vi "Omniax_mDrive_XY_MM_BR_RES.vi"() -> ()   [LabVIEW 2009]
uses:
  <vilib>/Instr/_visa.llb/VISA Configure Serial Port (Instr).vi
panel:
  out "Reset X Motor Steps":i32
  in  "Rese X Position mm":dbl
  out "X Backlash corr":bool
  out "X  in Motion":bool
  out "X Scan":bool
  out "X  in Range":bool
  out "X Step PV":i32 max=2000
  out "X Position mm PV":dbl
  out "X scan steps/sec MV step/sec":i32
  in  "X Scan set":bool
  in  "X Scan Velocity SP mm/sec":dbl
  in  "X Scan Length SP mm":dbl
  in  "X Move Set":bool
  out "X Velocity MV mm/sec":dbl
  in  "X Velocity SP mm/sec":dbl
  in  "X Position SP mm":dbl
  out "X Position MV mm":dbl
  out "X Scan velocity MV mm/sec":dbl format="%#_6f"
  out "X Scan length MV mm":dbl
  in  "X Scan Length SP steps":i32 min=-460800 max=460800 step=100
  in  "X Scan OK":bool
  in  "X Velocity SP step/sec":i32 min=1 max=102400
  in  "X Scan Velocity SP steps/sec":i32=1 min=1 max=102400 step=1
  in  "X Go":bool
  in  "X Step SP":i32=-20000 min=-460800 max=460800 step=500
  out "X Backlash steps/sec":i32
  out "X Backlash":i32
  out "X Holding Current %":i32
  out "X Run Current %":i32
  out "X offset mm":dbl
  out "X mm/rev":dbl
  out "X steps/rev":u32
  out "X MAXPOS":i32=-34296
  out "X MINPOS":i32=-94296
  out "X COM PORT":refnum<visa-resource-name>="COM5"
  out "Y Backlash corr":bool
  in  "Y Scan set":bool
  in  "Y Scan Velocity SP mm/sec":dbl
  in  "Y Scan Length SP mm":dbl
  in  "Y Move Set":bool
  out "Y Backlash steps/sec":i32
  out "Y Backlash":i32
  out "Y in Motion":bool
  in  "Reset":bool
  out "Reset Y Motor Steps":i32
  in  "Reset Y Position mm":dbl
  out "Y Velocity MV mm/sec":dbl
  in  "Y Velocity SP mm/sec":dbl
  in  "Y Position SP mm":dbl
  out "Y Position MV mm":dbl
  out "Y Holding Current %":i32
  out "Y Run Current %":i32
  out "Y Scan velocity MV mm/sec":dbl format="%#_6f"
  out "Y Scan length MV mm":dbl
  in  "Scan Cancel":bool
  out "Y Position mm PV":dbl
  out "Y offset mm":dbl
  out "Y mm/rev":dbl
  out "Y steps/rev":u32
  out "Y scan steps/sec MV step/sec":i32
  in  "Y Scan Length SP steps":i32 min=-460800 max=460800 step=100
  out "Y Scan":bool
  in  "Y Scan OK":bool
  in  "Scan Go":bool
  in  "Y Velocity SP step/sec":i32 min=1 max=102400
  in  "Y Scan Velocity SP steps/sec":i32=1 min=1 max=102400 step=1
  in  "Stop":bool
  out "Y in Range":bool
  out "Y Step PV":i32 max=2000
  in  "Y Go":bool
  in  "Y Step SP":i32=-20000 min=-460800 max=460800 step=500
  out "Y MINPOS":i32=-94296
  out "Y MAXPOS":i32=-34296
  out "Y COM PORT":refnum<visa-resource-name>="COM5"
  # "LM"
  # "MV"
  # "BL"
  # "SC"
  # "MX"
  # "MY"
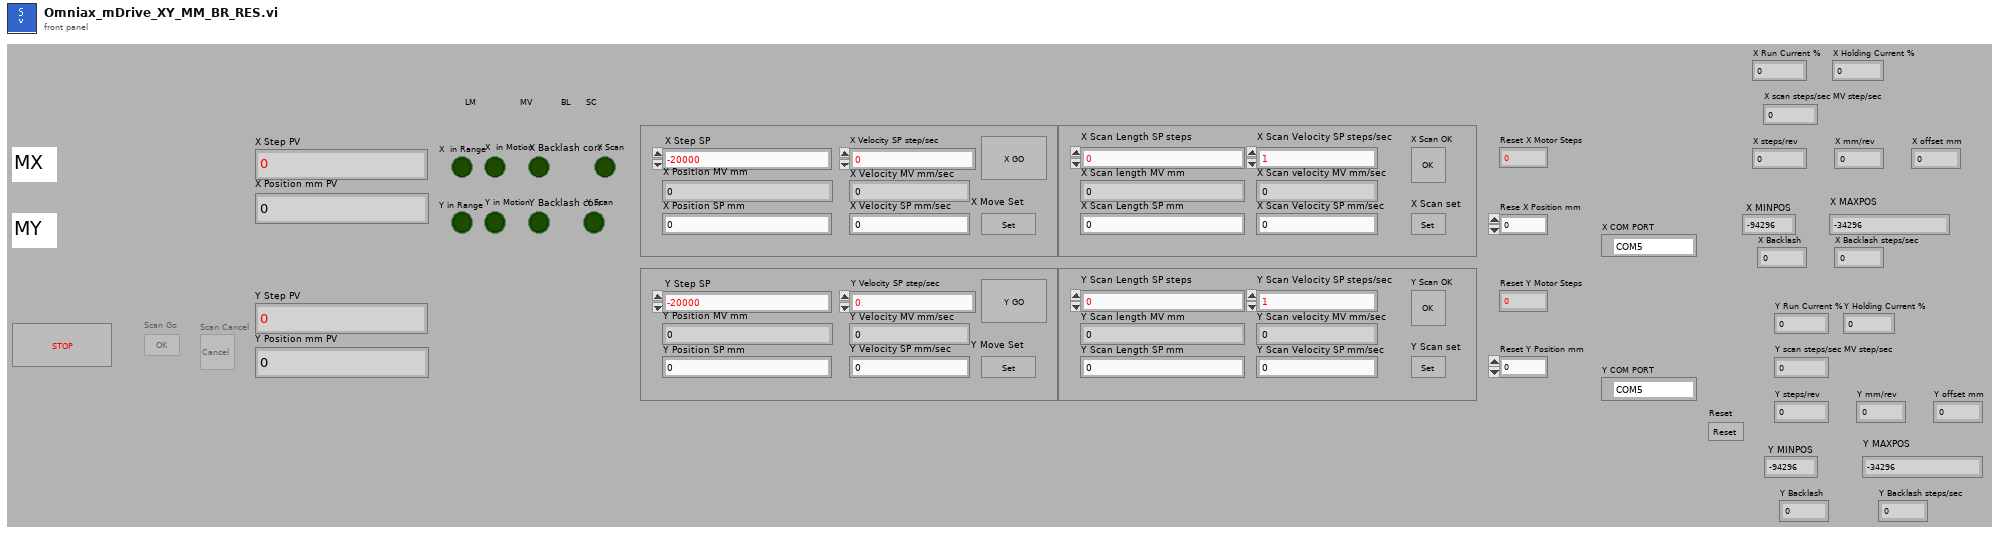
[diagram p1: front panel]
types:
  T1 = enum8{"Enabled", "Disabled", "Disabled and Grayed Out"}
  T2 = enum16{"Stop", "Reset", "Run Current", "Holding Current", "Accel Rate", "Decel Rate", "Move to Relative Position", "Move to Absolute Position", "Echo Mode", "Print Parameter", "Send String", "Microstep Resolution", "Set Current Position", "Max Velocity"}
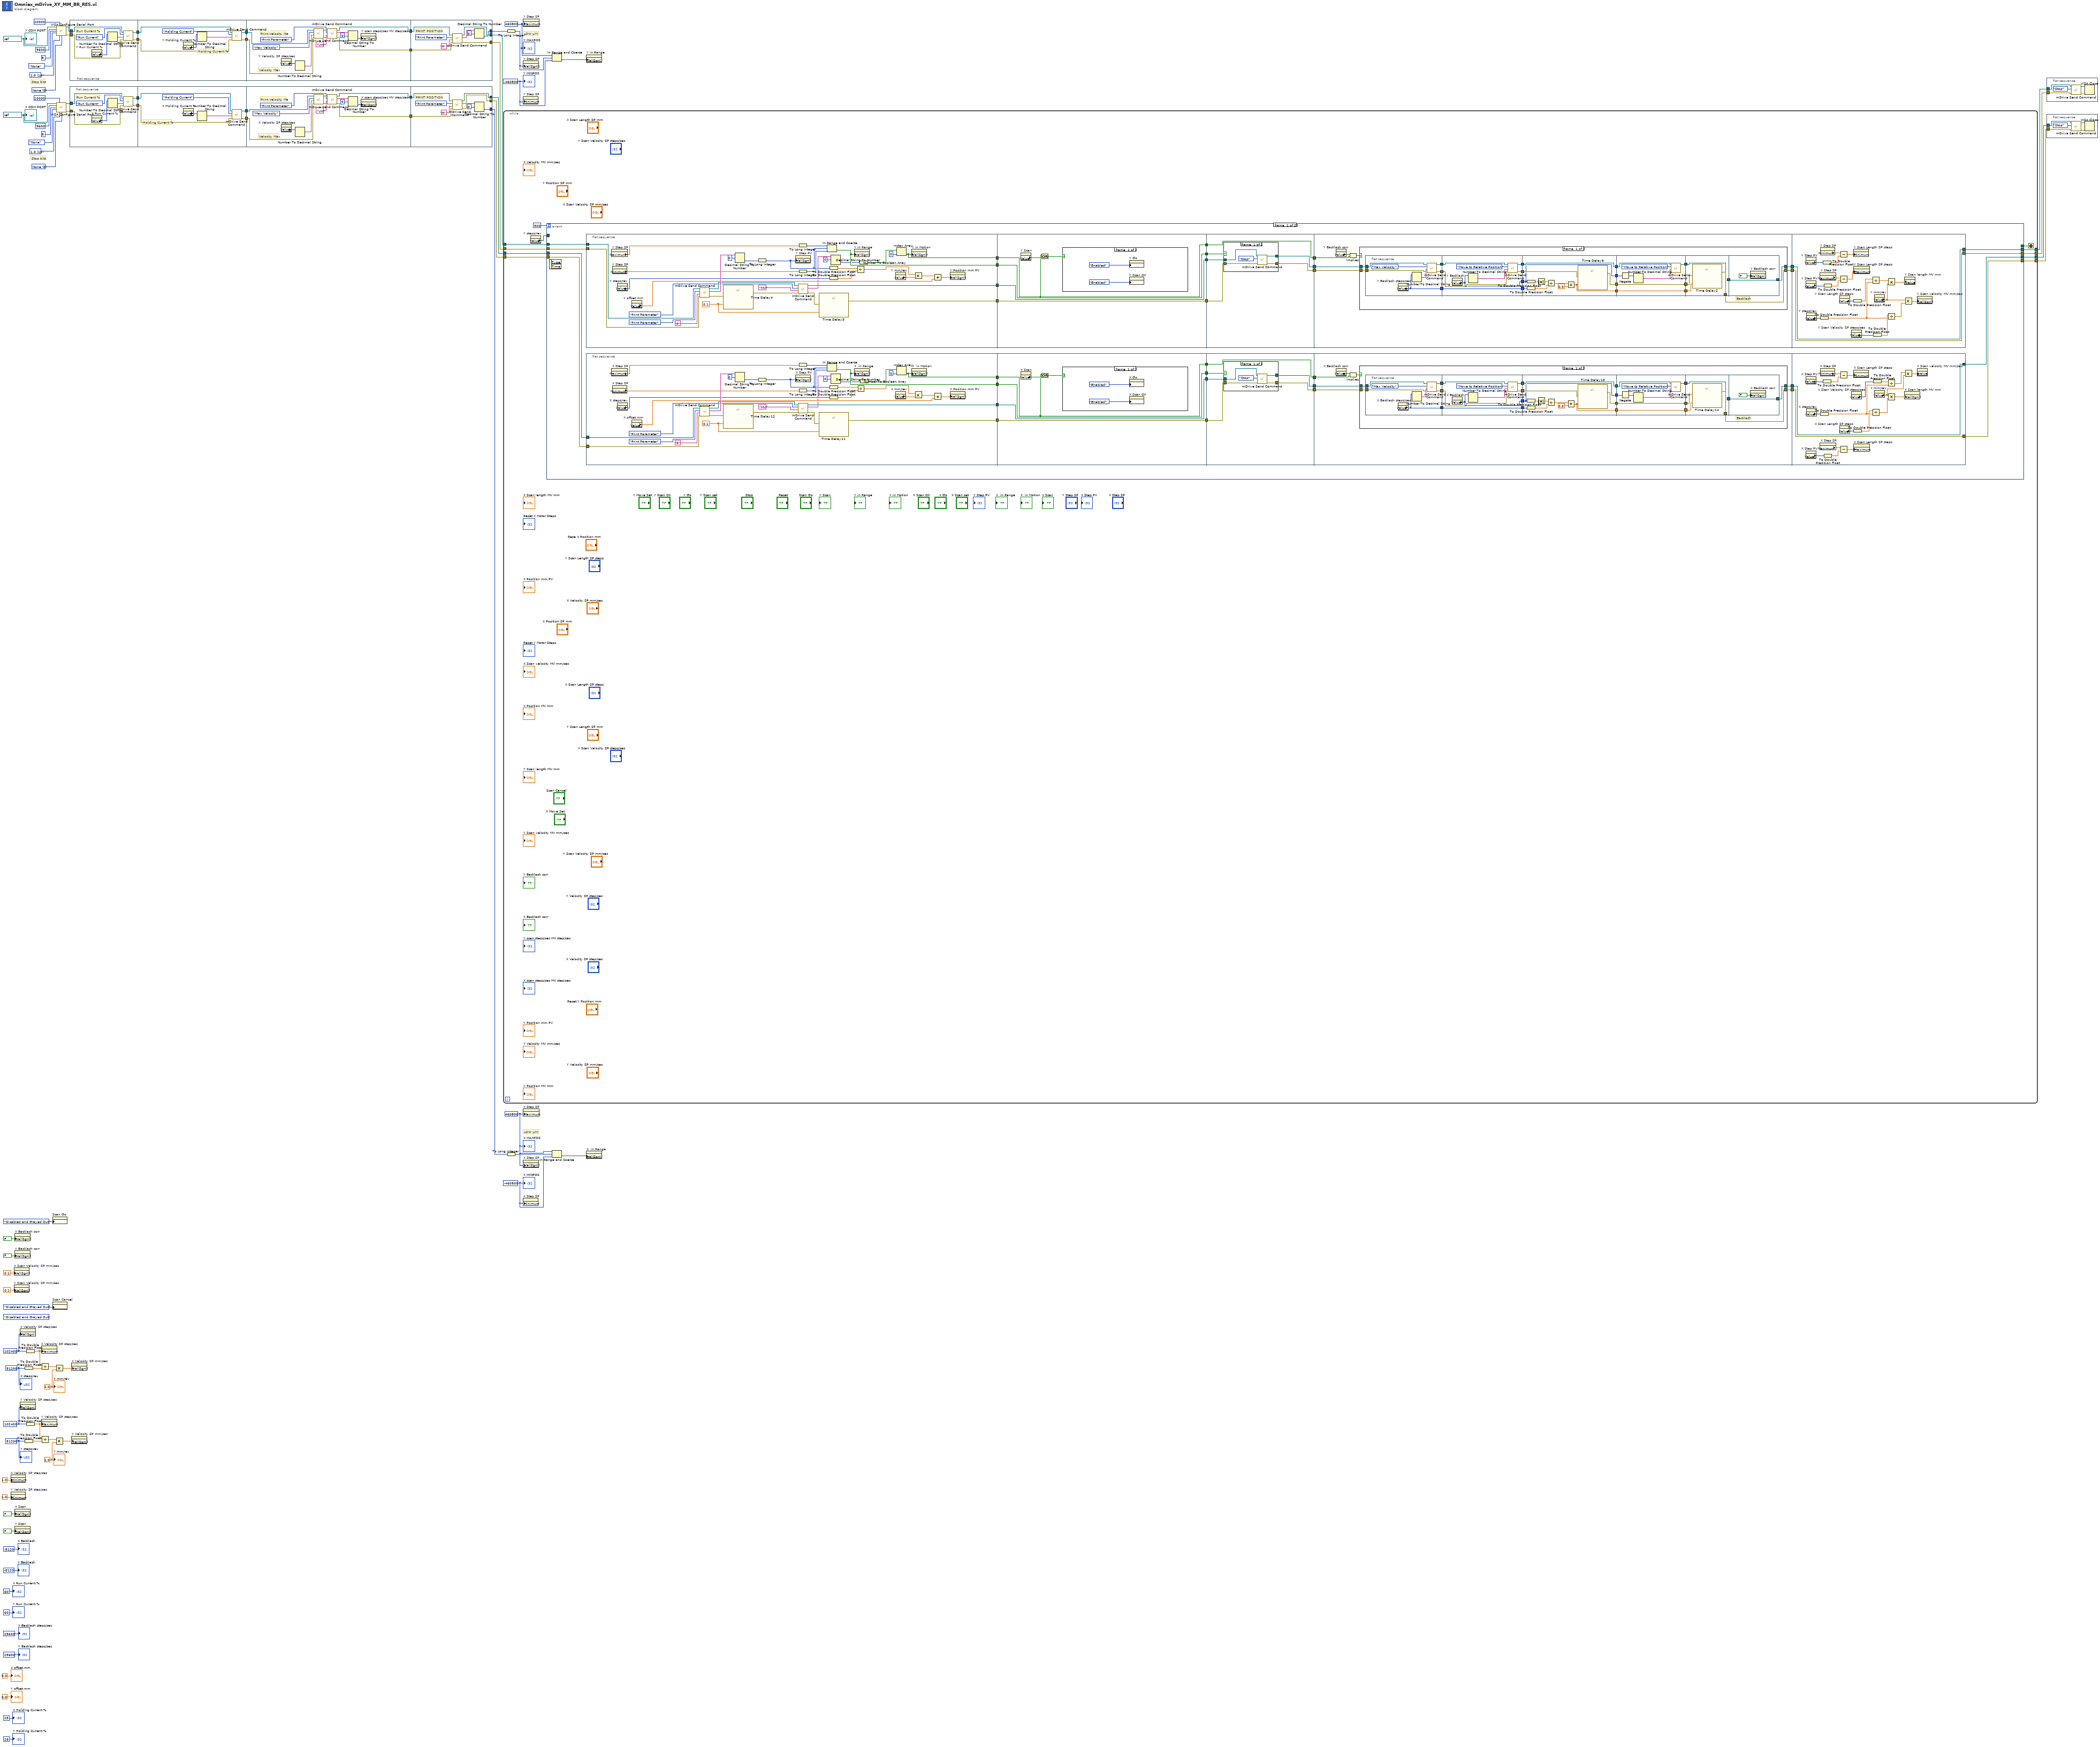
[diagram p0: block diagram]
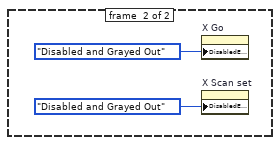
[diagram p2: hidden frame]
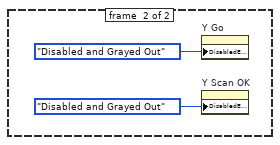
[diagram p5: hidden frame]
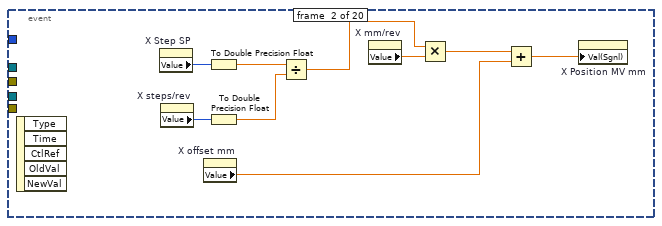
[diagram p8: hidden frame]
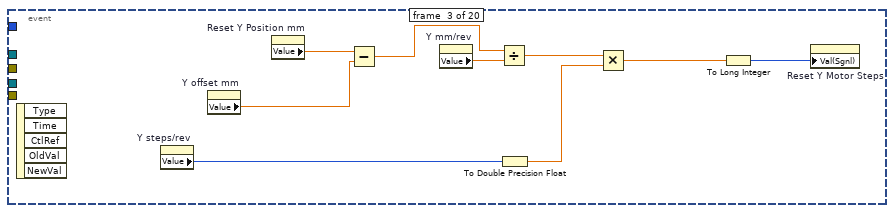
[diagram p9: hidden frame]
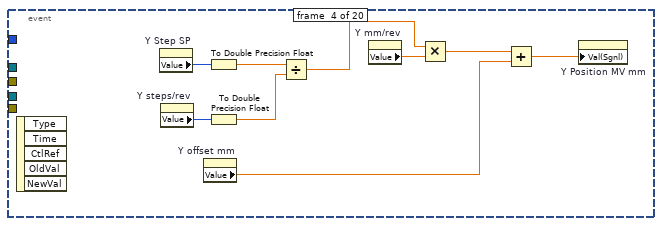
[diagram p10: hidden frame]
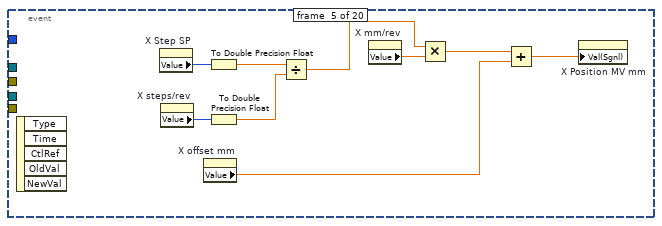
[diagram p11: hidden frame]
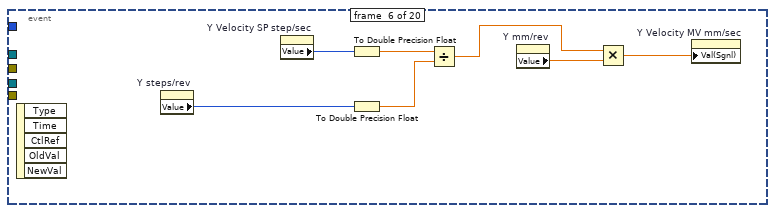
[diagram p12: hidden frame]
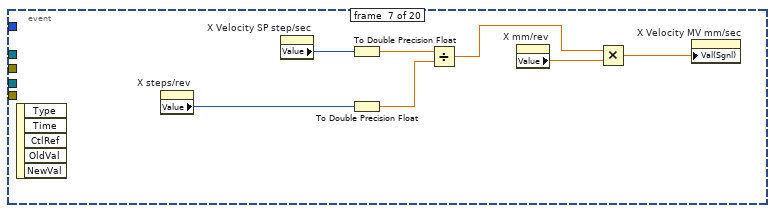
[diagram p13: hidden frame]
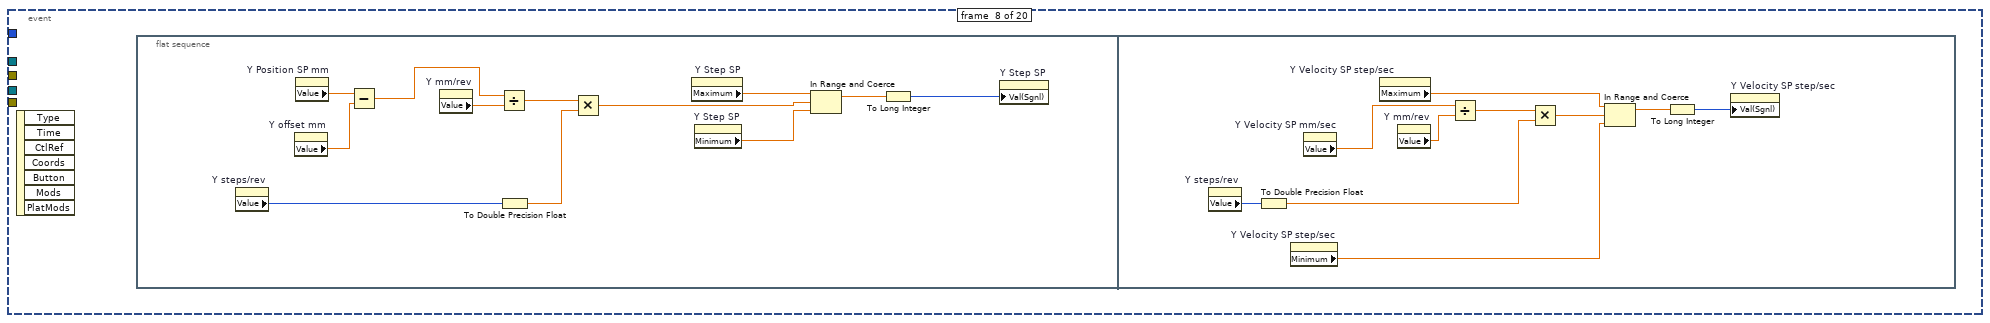
[diagram p14: hidden frame]
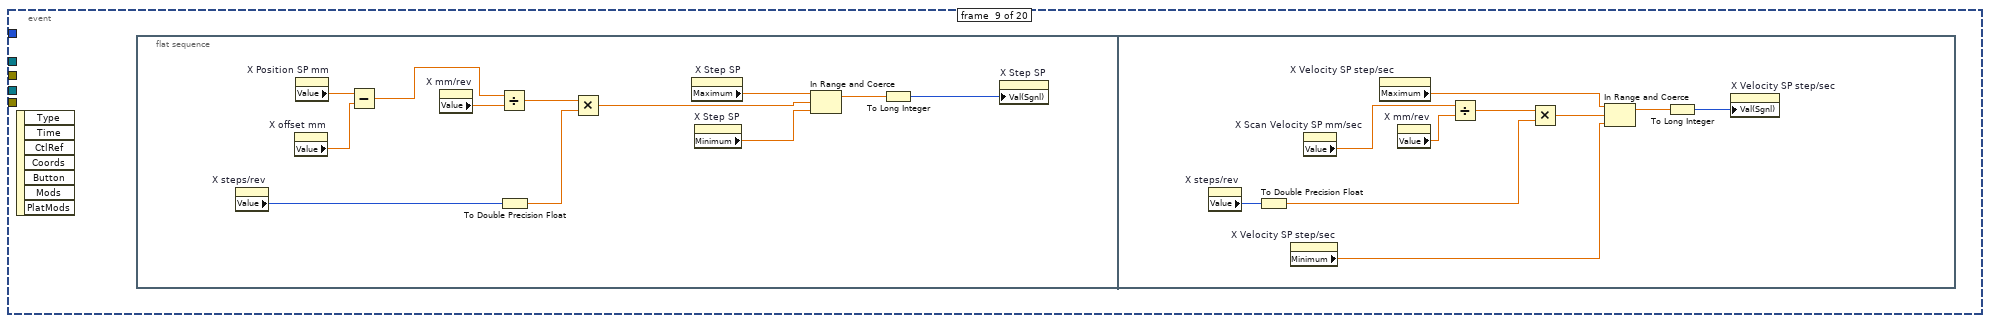
[diagram p15: hidden frame]
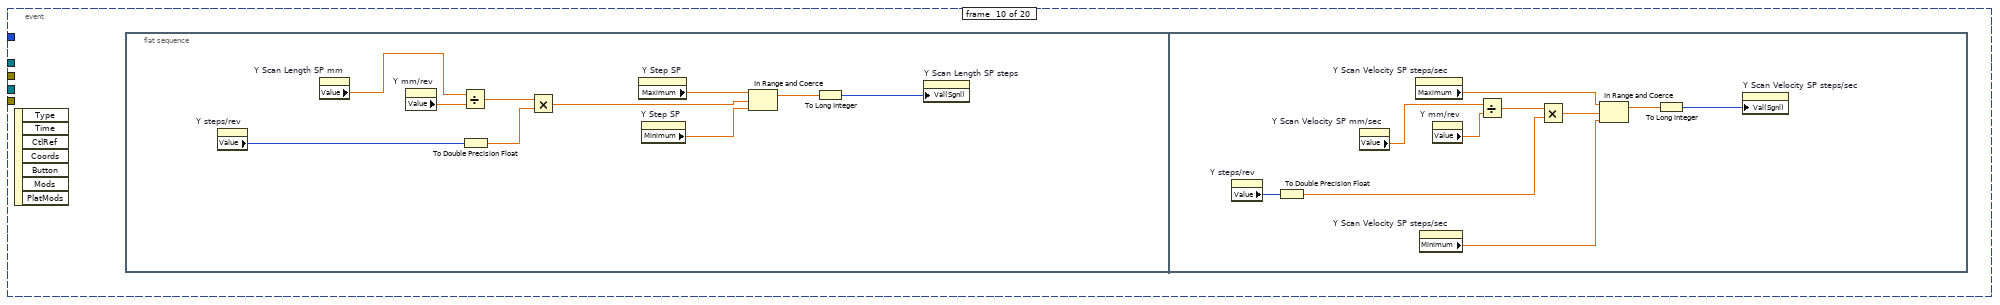
[diagram p16: hidden frame]
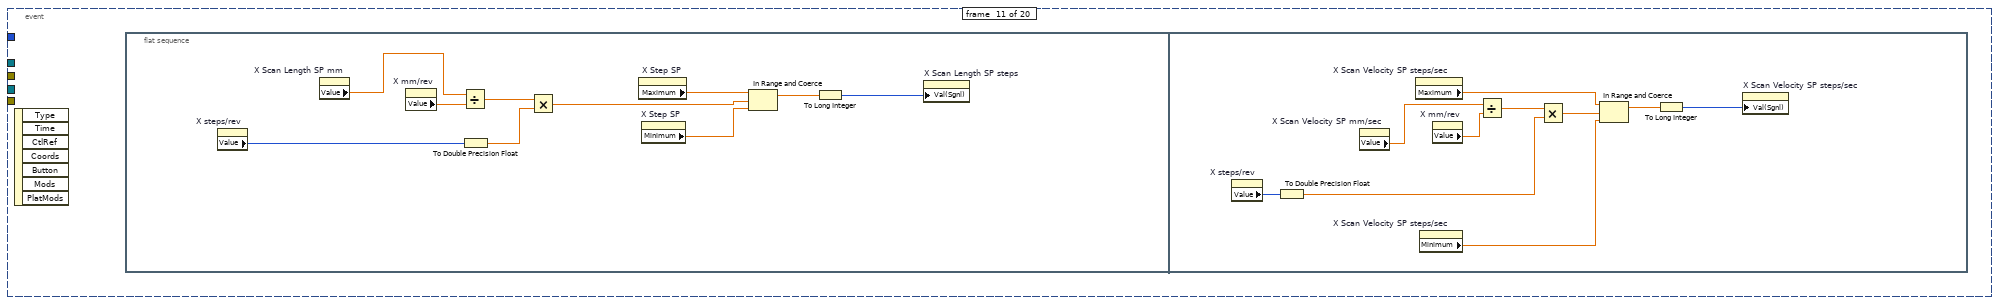
[diagram p17: hidden frame]
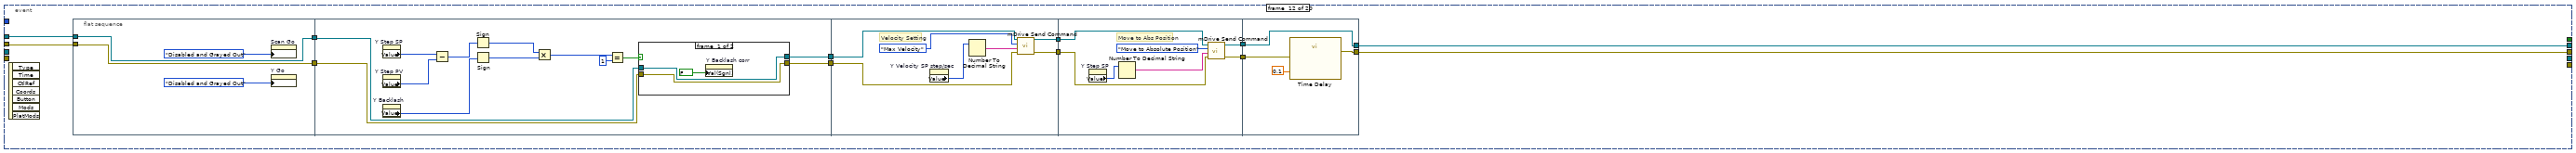
[diagram p18: hidden frame]
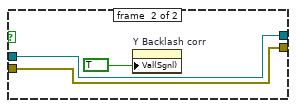
[diagram p19: hidden frame]
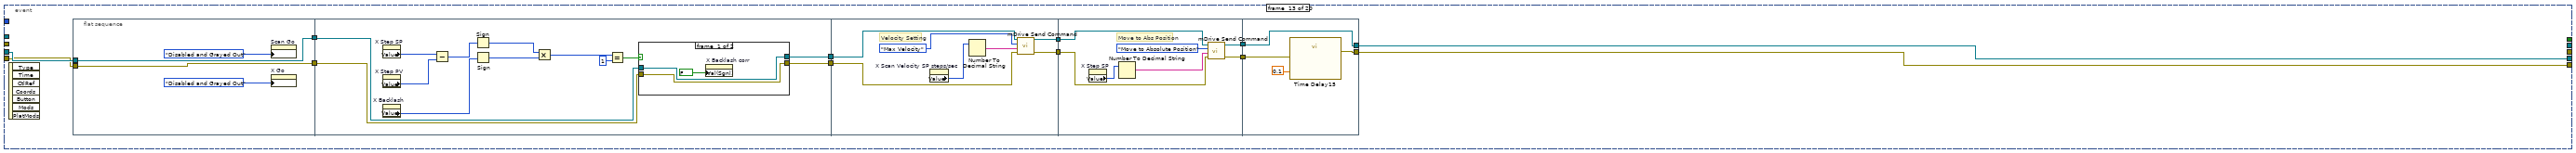
[diagram p20: hidden frame]
diagram:
  (unwired) T1."Disabled and Grayed Out" ("Disabled")
  w13 = 1.0 ("MM/rev")
  w10 = u32 51200 ("step/rev")
  w15 = 102400 ("Value (Signaling)")
  w25 = -460800 ("lower limit")
  w24 = 460800 ("upper limit")
  w28 = refnum<visa-resource-name> "COM8" ("COM PORT")
  w30 = u16 0 items=["None", "XON/XOFF", "RTS/CTS", "XON/XOFF & RTS/CTS", "DTR/DSR", "XON/XOFF & DTR/DSR"] ("flow control (0:none)")
  w31 = u16 10 items=["1.0"=10, "1.5"=15, "2.0"=20] ("stop bits (10: 1 bit)")
  w49 = 1.0 ("MM/rev")
  w46 = u32 51200 ("step/rev")
  w51 = 102400 ("Value (Signaling)")
  w69 = -460800 ("lower limit")
  w68 = 460800 ("upper limit")
  w76 = refnum<visa-resource-name> "COM9" ("COM PORT")
  w78 = u16 0 items=["None", "XON/XOFF", "RTS/CTS", "XON/XOFF & RTS/CTS", "DTR/DSR", "XON/XOFF & DTR/DSR"] ("flow control (0:none)")
  w79 = u16 10 items=["1.0"=10, "1.5"=15, "2.0"=20] ("stop bits (10: 1 bit)")
  # "LOW LIM"
  # "Stop bits"
  # "LOW LIM"
  # "Stop bits"
  n1 = property on="X Velocity SP step/sec" class="DigNum (strict)"("Minimum"=1.0 ("Data Entry Limits:Minimum")) -> ()  [unwired: 2 in, 2 out]
  n2 = property on="Y Velocity SP step/sec" class="DigNum (strict)"("Minimum"=1.0 ("Data Entry Limits:Minimum")) -> ()  [unwired: 2 in, 2 out]
  n3 = property on="X Scan Velocity SP mm/sec" class="DigNum (strict)"("Val(Sgnl)"=0.1 ("Value (Signaling)")) -> ()  [unwired: 2 in, 2 out]
  n4 = property on="Y Scan Velocity SP mm/sec" class="DigNum (strict)"("Val(Sgnl)"=0.1 ("Value (Signaling)")) -> ()  [unwired: 2 in, 2 out]
  n5 = property on="X Backlash corr" class="Bool (strict)"("Val(Sgnl)"=FALSE ("Value (Signaling)")) -> ()  [unwired: 2 in, 2 out]
  n6 = property on="Y Backlash corr" class="Bool (strict)"("Val(Sgnl)"=FALSE ("Value (Signaling)")) -> ()  [unwired: 2 in, 2 out]
  n7 = property on="X Scan" class="Bool (strict)"("Val(Sgnl)"=FALSE ("Value (Signaling)")) -> ()  [unwired: 2 in, 2 out]
  n8 = property on="Y Scan" class="Bool (strict)"("Val(Sgnl)"=FALSE ("Value (Signaling)")) -> ()  [unwired: 2 in, 2 out]
  n9 = property on="X Velocity SP step/sec" class="DigNum (strict)"("Val(Sgnl)"=w15) -> ()  [unwired: 2 in, 2 out]
  n10 = property on="Y Velocity SP step/sec" class="DigNum (strict)"("Val(Sgnl)"=w51) -> ()  [unwired: 2 in, 2 out]
  n11 = To Double Precision Float(number=w10) -> (double precision float=w11:dbl)
  n12 = To Double Precision Float(number=w46) -> (double precision float=w47:dbl)
  n13 = To Double Precision Float(number=w15) -> (double precision float=w9:dbl)
  n14 = To Double Precision Float(number=w51) -> (double precision float=w45:dbl)
  n15 = Divide(x=w9, y=w11) -> (x/y=w14:dbl)
  n16 = Divide(x=w45, y=w47) -> (x/y=w50:dbl)
  n17 = property on="X Velocity SP step/sec" class="DigNum (strict)"("Maximum"=w9) -> ()  [unwired: 2 in, 2 out]
  n18 = property on="Y Velocity SP step/sec" class="DigNum (strict)"("Maximum"=w45) -> ()  [unwired: 2 in, 2 out]
  n19 = property on="Scan Go" class="Bool"("DisabledEnum"=T1."Disabled and Grayed Out" ("Disabled")) -> ()  [unwired: 2 in, 2 out]
  n20 = property on="Scan Cancel" class="Bool"("DisabledEnum"=T1."Disabled and Grayed Out" ("Disabled")) -> ()  [unwired: 2 in, 2 out]
  n21 = Multiply(x=w14, y=w13) -> (x*y=w12:dbl)
  n22 = Multiply(x=w50, y=w49) -> (x*y=w48:dbl)
  n23 = call-poly "VISA Configure Serial Port"("VISA resource name"=w76, "timeout (10sec)"=u32 10000, "baud rate (9600)"=u32 9600, "data bits (8)"=u16 8, "parity (0:none)"=enum16{"None", "Odd", "Even", "Mark", "Space"}."None", "stop bits (10: 1 bit)"=w79, "flow control (0:none)"=w78) -> ("VISA resource name out"=w64:refnum<visa-resource-name>, "error out"=w63:errorcluster)  [unwired: 7 in]
  n24 = call-poly "VISA Configure Serial Port"("VISA resource name"=w28, "timeout (10sec)"=u32 10000, "baud rate (9600)"=u32 9600, "data bits (8)"=u16 8, "parity (0:none)"=enum16{"None", "Odd", "Even", "Mark", "Space"}."None", "stop bits (10: 1 bit)"=w31, "flow control (0:none)"=w30) -> ("VISA resource name out"=w22:refnum<visa-resource-name>, "error out"=w21:errorcluster)  [unwired: 7 in]
  n25 = flat-sequence {
    tunnel: w63 -> [w89]
    tunnel: w64 -> [w87]
    tunnel: [w86] -> w58
    tunnel: [w88] -> w56
    tunnel: w58 -> [w96]
    tunnel: [w95] -> w57
    tunnel: w56 -> [w93]
    tunnel: [w94] -> w55
    tunnel: [w106] -> w66
    tunnel: [w107] -> w65
    tunnel: w57 -> [w105]
    tunnel: w55 -> [w104]
    tunnel: [w119] -> w75
    tunnel: [w118] -> w74
    tunnel: [w113] -> w67
    tunnel: w66 -> [w117]
    tunnel: w65 -> [w116]
    frame #0 {
      # "Run Current %"
      n26 = property on="Y Run Current %" class="DigNum (strict)"() -> ("Value"=w84:i32)  [unwired: 2 in, 2 out]
      n27 = Number To Decimal String(number=w84) -> (decimal integer string=w85:string)  [unwired: 1 in]
      n28 = call "mDrive Send Command.vi"("error in (no error)"=w89, "Extra"=w85, "Command"=T2."Run Current", "VISA resource name"=w87) -> ("error out"=w88:errorcluster, "VISA resource name out"=w86:refnum<visa-resource-name>)  [unwired: 3 in, 1 out]
    }
    frame #1 {
      # "Holding Current %"
      n29 = property on="Y Holding Current %" class="DigNum (strict)"() -> ("Value"=w91:i32)  [unwired: 2 in, 2 out]
      n30 = Number To Decimal String(number=w91) -> (decimal integer string=w92:string)  [unwired: 1 in]
      n31 = call "mDrive Send Command.vi"("error in (no error)"=w93, "Extra"=w92, "Command"=T2."Holding Current", "VISA resource name"=w96) -> ("error out"=w94:errorcluster, "VISA resource name out"=w95:refnum<visa-resource-name>)  [unwired: 3 in, 1 out]
    }
    frame #2 {
      # "Print Velocity Ma"
      # "Velocity Max"
      n32 = property on="Y Velocity SP step/sec" class="DigNum (strict)"() -> ("Value"=w103:i32)  [unwired: 2 in, 2 out]
      n33 = Number To Decimal String(number=w103) -> (decimal integer string=w102:string)  [unwired: 1 in]
      n34 = call "mDrive Send Command.vi"("error in (no error)"=w104, "Extra"=w102, "Command"=T2."Max Velocity", "VISA resource name"=w105) -> ("error out"=w100:errorcluster, "VISA resource name out"=w110:refnum<visa-resource-name>)  [unwired: 3 in, 1 out]
      n35 = call "mDrive Send Command.vi"("error in (no error)"=w100, "Extra"="VM", "Command"=T2."Print Parameter", "VISA resource name"=w110) -> ("error out"=w107:errorcluster, "read buffer"=w108:string, "VISA resource name out"=w106:refnum<visa-resource-name>)  [unwired: 3 in]
      n36 = Decimal String To Number(string=w108, offset=0) -> (number=w101:i32)  [unwired: 1 in, 1 out]
      n37 = property on="Y scan steps/sec MV step/sec" class="DigNum (strict)"("Val(Sgnl)"=w101) -> ()  [unwired: 2 in, 2 out]
    }
    frame #3 {
      # "PRINT POSITION"
      n38 = call "mDrive Send Command.vi"("error in (no error)"=w116, "Extra"="P", "Command"=T2."Print Parameter", "VISA resource name"=w117) -> ("error out"=w118:errorcluster, "read buffer"=w115:string, "VISA resource name out"=w119:refnum<visa-resource-name>)  [unwired: 3 in]
      n39 = Decimal String To Number(string=w115, offset=0) -> (number=w113:i32)  [unwired: 1 in, 1 out]
    }
  }
  n40 = flat-sequence {
    tunnel: w21 -> [w126]
    tunnel: w22 -> [w124]
    tunnel: [w123] -> w40
    tunnel: [w125] -> w39
    tunnel: w40 -> [w133]
    tunnel: [w132] -> w38
    tunnel: w39 -> [w130]
    tunnel: [w131] -> w37
    tunnel: [w143] -> w36
    tunnel: [w144] -> w35
    tunnel: w38 -> [w142]
    tunnel: w37 -> [w141]
    tunnel: [w156] -> w4
    tunnel: [w155] -> w3
    tunnel: [w150] -> w23
    tunnel: w36 -> [w154]
    tunnel: w35 -> [w153]
    frame #0 {
      # "Run Current %"
      n41 = property on="X Run Current %" class="DigNum (strict)"() -> ("Value"=w121:i32)  [unwired: 2 in, 2 out]
      n42 = Number To Decimal String(number=w121) -> (decimal integer string=w122:string)  [unwired: 1 in]
      n43 = call "mDrive Send Command.vi"("error in (no error)"=w126, "Extra"=w122, "Command"=T2."Run Current", "VISA resource name"=w124) -> ("error out"=w125:errorcluster, "VISA resource name out"=w123:refnum<visa-resource-name>)  [unwired: 3 in, 1 out]
    }
    frame #1 {
      # "Holding Current %"
      n44 = property on="X Holding Current %" class="DigNum (strict)"() -> ("Value"=w128:i32)  [unwired: 2 in, 2 out]
      n45 = Number To Decimal String(number=w128) -> (decimal integer string=w129:string)  [unwired: 1 in]
      n46 = call "mDrive Send Command.vi"("error in (no error)"=w130, "Extra"=w129, "Command"=T2."Holding Current", "VISA resource name"=w133) -> ("error out"=w131:errorcluster, "VISA resource name out"=w132:refnum<visa-resource-name>)  [unwired: 3 in, 1 out]
    }
    frame #2 {
      # "Print Velocity Ma"
      # "Velocity Max"
      n47 = property on="X Velocity SP step/sec" class="DigNum (strict)"() -> ("Value"=w140:i32)  [unwired: 2 in, 2 out]
      n48 = Number To Decimal String(number=w140) -> (decimal integer string=w139:string)  [unwired: 1 in]
      n49 = call "mDrive Send Command.vi"("error in (no error)"=w141, "Extra"=w139, "Command"=T2."Max Velocity", "VISA resource name"=w142) -> ("error out"=w137:errorcluster, "VISA resource name out"=w147:refnum<visa-resource-name>)  [unwired: 3 in, 1 out]
      n50 = call "mDrive Send Command.vi"("error in (no error)"=w137, "Extra"="VM", "Command"=T2."Print Parameter", "VISA resource name"=w147) -> ("error out"=w144:errorcluster, "read buffer"=w145:string, "VISA resource name out"=w143:refnum<visa-resource-name>)  [unwired: 3 in]
      n51 = Decimal String To Number(string=w145, offset=0) -> (number=w138:i32)  [unwired: 1 in, 1 out]
      n52 = property on="X scan steps/sec MV step/sec" class="DigNum (strict)"("Val(Sgnl)"=w138) -> ()  [unwired: 2 in, 2 out]
    }
    frame #3 {
      # "PRINT POSITION"
      n53 = call "mDrive Send Command.vi"("error in (no error)"=w153, "Extra"="P", "Command"=T2."Print Parameter", "VISA resource name"=w154) -> ("error out"=w155:errorcluster, "read buffer"=w152:string, "VISA resource name out"=w156:refnum<visa-resource-name>)  [unwired: 3 in]
      n54 = Decimal String To Number(string=w152, offset=0) -> (number=w150:i32)  [unwired: 1 in, 1 out]
    }
  }
  n55 = property on="X Velocity SP mm/sec" class="DigNum (strict)"("Val(Sgnl)"=w12) -> ()  [unwired: 2 in, 2 out]
  n56 = property on="Y Velocity SP mm/sec" class="DigNum (strict)"("Val(Sgnl)"=w48) -> ()  [unwired: 2 in, 2 out]
  n57 = while {
    tunnel: w75 -> [w163]
    tunnel: w74 -> [w166]
    tunnel: [w167] -> w71
    tunnel: [w165] -> w72
    tunnel: w4 -> [w160]
    tunnel: w3 -> [w159]
    tunnel: [w158] -> w2
    tunnel: [w157] -> w1
    stop <- w162 stop-if-true
    n58 = property on="Y steps/rev" class="DigNum (strict)"() -> ("Value"=w161:u32)  [unwired: 2 in, 2 out]
    n59 = event shown="[18] \"Scan Go\": Mouse Up" {
      selector: _ -> [_ _ _ _ _ _ _ _ _ _ _ _ _ _ _ _ _ _ _ _]
      dyn-events: _ -> [_ _ _ _ _ _ _ _ _ _ _ _ _ _ _ _ _ _ _ _]
      timeout: 500 -> [_ _ _ _ _ _ _ _ _ _ _ _ _ _ _ _ _ _ _ _]
      tunnel: w166 -> [w201 _ _ _ _ _ _ _ _ _ _ w636 _ _ w780 w809 w819 w831 w877 w933]
      tunnel: [w200 _ _ _ _ _ _ _ _ _ _ w642 _ _ w778 w809 w817 w833 w874 w931] -> w167
      tunnel: w163 -> [w198 _ _ _ _ _ _ _ _ _ _ w637 _ _ w779 w810 w820 w832 w876 w934]
      tunnel: [w199 _ _ _ _ _ _ _ _ _ _ w643 _ _ w775 w810 w818 w834 w875 w932] -> w165
      tunnel: [_ _ _ _ _ _ _ _ _ _ _ _ _ _ _ TRUE _ _ _ _] -> w162
      tunnel: w161 -> [_ _ _ _ _ _ _ _ _ _ _ _ _ _ _ _ _ _ _ _]
      tunnel: w160 -> [w171 _ _ _ _ _ _ _ _ _ _ _ w688 w743 _ _ w812 w824 _ w930]
      tunnel: w159 -> [w170 _ _ _ _ _ _ _ _ _ _ _ w687 w742 _ _ w811 w823 _ w929]
      tunnel: [w169 _ _ _ _ _ _ _ _ _ _ _ w686 w741 _ _ w814 w822 _ w928] -> w158
      tunnel: [w168 _ _ _ _ _ _ _ _ _ _ _ w685 w740 _ _ w813 w821 _ w927] -> w157
      event #0 {
        n60 = event-data() -> ()  [unwired: 1 in, 2 out]
        n61 = flat-sequence {
          tunnel: w201 -> [w380]
          tunnel: w198 -> [w379]
          tunnel: [w385] -> w197
          tunnel: [w359] -> w195
          tunnel: [w372] -> w193
          tunnel: [w350] -> w191
          tunnel: w197 -> [w391]
          tunnel: [w391] -> w196
          tunnel: w195 -> [w390]
          tunnel: [w390] -> w194
          tunnel: w193 -> [w389]
          tunnel: [w389] -> w192
          tunnel: w191 -> [w386]
          tunnel: [w386] -> w186
          tunnel: w196 -> [w398]
          tunnel: [w399] -> w190
          tunnel: w194 -> [w401]
          tunnel: [w400] -> w189
          tunnel: w192 -> [w397]
          tunnel: [w396] -> w187
          tunnel: w186 -> [w396]
          tunnel: w190 -> [w411]
          tunnel: w189 -> [w412]
          tunnel: [w410] -> w188
          tunnel: w187 -> [w414]
          tunnel: [w409] -> w185
          tunnel: [w496] -> w200
          tunnel: [w497] -> w199
          tunnel: w188 -> [w496]
          tunnel: w185 -> [w497]
          frame #0 {
            w354 = 0.1 ("Delay Time (s)")
            n62 = property on="Y Step SP" class="DigNum (strict)"() -> ("Maximum"=w374:dbl)  [unwired: 2 in, 2 out]
            n63 = property on="Y Step SP" class="DigNum (strict)"() -> ("Minimum"=w376:dbl)  [unwired: 2 in, 2 out]
            n64 = property on="Y steps/rev" class="DigNum (strict)"() -> ("Value"=w370:u32)  [unwired: 2 in, 2 out]
            n65 = property on="Y offset mm" class="DigNum (strict)"() -> ("Value"=w366:dbl)  [unwired: 2 in, 2 out]
            n66 = call "mDrive Send Command.vi"("error in (no error)"=w380, "Extra"="P", "Command"=T2."Print Parameter", "VISA resource name"=w379) -> ("error out"=w378:errorcluster, "read buffer"=w384:string, "VISA resource name out"=w382:refnum<visa-resource-name>)  [unwired: 3 in]
            n67 = call "Time Delay4"("error in (no error)"=w378, "Delay Time (s)"=w354) -> ("error out"=w377:errorcluster)  [unwired: 9 in]
            n68 = Decimal String To Number(string=w384, offset=0) -> (number=w362:i32)  [unwired: 1 in, 1 out]
            n69 = To Long Integer(number=w362) -> (32bit integer=w364:i32)
            n70 = property on="Y Step PV" class="DigNum (strict)"("Val(Sgnl)"=w364) -> ()  [unwired: 2 in, 2 out]
            n71 = To Long Integer(number=w374) -> (32bit integer=w373:i32)
            n72 = To Long Integer(number=w376) -> (32bit integer=w375:i32)
            n73 = call "mDrive Send Command.vi"("error in (no error)"=w377, "Extra"="MV", "Command"=T2."Print Parameter", "VISA resource name"=w382) -> ("error out"=w381:errorcluster, "read buffer"=w360:string, "VISA resource name out"=w385:refnum<visa-resource-name>)  [unwired: 3 in]
            n74 = call "Time Delay3"("error in (no error)"=w381, "Delay Time (s)"=w354) -> ("error out"=w359:errorcluster)  [unwired: 9 in]
            n75 = In Range and Coerce(upper limit=w373, x=w364, lower limit=w375) -> (In Range?=w372:bool)  [unwired: 1 out]
            n76 = To Double Precision Float(number=w364) -> (double precision float=w365:dbl)
            n77 = To Double Precision Float(number=w370) -> (double precision float=w371:dbl)
            n78 = Decimal String To Number(string=w360, offset=0 ("offset (0)")) -> (number=w353:i32)  [unwired: 1 in, 1 out]
            n79 = property on="Y in Range" class="Bool (strict)"("Val(Sgnl)"=w372) -> ()  [unwired: 2 in, 2 out]
            n80 = Divide(x=w365, y=w371) -> (x/y=w369:dbl)
            n81 = Number To Boolean Array(number=w353) -> (Boolean array=w352:bool[])
            n82 = property on="Y mm/rev" class="DigNum (strict)"() -> ("Value"=w368:dbl)  [unwired: 2 in, 2 out]
            n83 = Index Array(array=w352, index=0) -> (element=w350:bool)
            n84 = property on="Y in Motion" class="Bool (strict)"("Val(Sgnl)"=w350) -> ()  [unwired: 2 in, 2 out]
            n85 = Multiply(x=w369, y=w368) -> (x*y=w367:dbl)
            n86 = Add(x=w367, y=w366) -> (x+y=w363:dbl)
            n87 = property on="Y Position mm PV" class="DigNum (strict)"("Val(Sgnl)"=w363) -> ()  [unwired: 2 in, 2 out]
          }
          frame #1 {
            n88 = property on="Y Scan" class="Bool (strict)"() -> ("Value"=w387:bool)  [unwired: 2 in, 2 out]
            n89 = Or(x=w386, y=w387) -> (x .or. y?=w388:bool)
            n90 = case shown="False" w388 {
              frame #0 {
                n91 = property on="Y Go" class="Bool"("DisabledEnum"=T1."Enabled" ("Disabled")) -> ()  [unwired: 2 in, 2 out]
                n92 = property on="Y Scan OK" class="Bool"("DisabledEnum"=T1."Enabled" ("Disabled")) -> ()  [unwired: 2 in, 2 out]
              }
              frame #1 {
                n93 = property on="Y Go" class="Bool"("DisabledEnum"=T1."Disabled and Grayed Out" ("Disabled")) -> ()  [unwired: 2 in, 2 out]
                n94 = property on="Y Scan OK" class="Bool"("DisabledEnum"=T1."Disabled and Grayed Out" ("Disabled")) -> ()  [unwired: 2 in, 2 out]
              }
            }
          }
          frame #2 {
            n95 = case shown="False" w397 {
              tunnel: w398 -> [w404 w408]
              tunnel: [w405 w408] -> w399
              tunnel: [w406 w407] -> w400
              tunnel: w401 -> [w403 w407]
              frame #0 {
                n96 = call "mDrive Send Command.vi"("error in (no error)"=w403, "Command"=T2."Stop", "VISA resource name"=w404) -> ("error out"=w406:errorcluster, "VISA resource name out"=w405:refnum<visa-resource-name>)  [unwired: 4 in, 1 out]
              }
              frame #1 {
              }
            }
          }
          frame #3 {
            n97 = property on="Y Backlash corr" class="Bool (strict)"() -> ("Value"=w415:bool)  [unwired: 2 in, 2 out]
            n98 = Implies(1:w414, 2:w415) -> (0:w413:bool)
            n99 = case shown="False" w413 {
              tunnel: w412 -> [w422 w475]
              tunnel: w411 -> [w421 w476]
              tunnel: [w420 w475] -> w410
              tunnel: [w419 w476] -> w409
              frame #0 {
                # "Backlash"
                n100 = flat-sequence {
                  tunnel: [w437] -> w434
                  tunnel: [w439] -> w433
                  tunnel: [w438] -> w432
                  tunnel: w422 -> [w436]
                  tunnel: w421 -> [w435]
                  tunnel: w434 -> [w447]
                  tunnel: [w447] -> w431
                  tunnel: w433 -> [w446]
                  tunnel: w432 -> [w445]
                  tunnel: [w444] -> w430
                  tunnel: [w443] -> w429
                  tunnel: [w442] -> w418
                  tunnel: w431 -> [w457]
                  tunnel: w430 -> [w456]
                  tunnel: w429 -> [w454]
                  tunnel: [w455] -> w428
                  tunnel: [w454] -> w427
                  tunnel: [w453] -> w424
                  tunnel: [w452] -> w423
                  tunnel: w418 -> [w452]
                  tunnel: w428 -> [w468]
                  tunnel: w427 -> [w461]
                  tunnel: [w468] -> w426
                  tunnel: [w467] -> w425
                  tunnel: w424 -> [w467]
                  tunnel: w423 -> [w463]
                  tunnel: [w462] -> w416
                  tunnel: w426 -> [w472]
                  tunnel: w425 -> [w471]
                  tunnel: [w470] -> w420
                  tunnel: [w469] -> w417
                  tunnel: w416 -> [w469]
                  tunnel: [w474] -> w419
                  tunnel: w417 -> [w474]
                  frame #0 {
                    n101 = property on="Y Backlash steps/sec" class="DigNum (strict)"() -> ("Value"=w437:i32)  [unwired: 2 in, 2 out]
                    n102 = Number To Decimal String(number=w437) -> (decimal integer string=w440:string)  [unwired: 1 in]
                    n103 = call "mDrive Send Command.vi"("error in (no error)"=w436, "Extra"=w440, "Command"=T2."Max Velocity", "VISA resource name"=w435) -> ("error out"=w438:errorcluster, "VISA resource name out"=w439:refnum<visa-resource-name>)  [unwired: 3 in, 1 out]
                  }
                  frame #1 {
                    n104 = property on="Y Backlash" class="DigNum (strict)"() -> ("Value"=w442:i32)  [unwired: 2 in, 2 out]
                    n105 = Number To Decimal String(number=w442) -> (decimal integer string=w448:string)  [unwired: 1 in]
                    n106 = call "mDrive Send Command.vi"("error in (no error)"=w445, "Extra"=w448, "Command"=T2."Move to Relative Position", "VISA resource name"=w446) -> ("error out"=w444:errorcluster, "VISA resource name out"=w443:refnum<visa-resource-name>)  [unwired: 3 in, 1 out]
                  }
                  frame #2 {
                    n107 = To Double Precision Float(number=w452) -> (double precision float=w450:dbl)
                    n108 = To Double Precision Float(number=w457) -> (double precision float=w459:dbl)
                    n109 = Absolute Value(x=w450) -> (abs(x)=w451:dbl)
                    n110 = Divide(x=w451, y=w459) -> (x/y=w460:dbl)
                    n111 = Add(x=w460, y=0.3) -> (x+y=w453:dbl)
                    n112 = call "Time Delay8"("error in (no error)"=w456, "Delay Time (s)"=w453) -> ("error out"=w455:errorcluster)  [unwired: 9 in]
                  }
                  frame #3 {
                    n113 = Negate(x=w463) -> (-x=w464:i32)
                    n114 = Number To Decimal String(number=w464) -> (decimal integer string=w465:string)  [unwired: 1 in]
                    n115 = call "mDrive Send Command.vi"("Extra"=w465, "Command"=T2."Move to Relative Position", "VISA resource name"=w461) -> ("VISA resource name out"=w462:refnum<visa-resource-name>)  [unwired: 4 in, 2 out]
                  }
                  frame #4 {
                    n116 = call "Time Delay2"("error in (no error)"=w472, "Delay Time (s)"=w471) -> ("error out"=w470:errorcluster)  [unwired: 9 in]
                  }
                  frame #5 {
                    n117 = property on="Y Backlash corr" class="Bool (strict)"("Val(Sgnl)"=FALSE ("Value (Signaling)")) -> ()  [unwired: 2 in, 2 out]
                  }
                }
              }
              frame #1 {
              }
            }
          }
          frame #4 {
            n118 = property on="Y Step PV" class="DigNum (strict)"() -> ("Value"=w484:i32)  [unwired: 2 in, 2 out]
            n119 = property on="Y Step PV" class="DigNum (strict)"() -> ("Value"=w486:i32)  [unwired: 2 in, 2 out]
            n120 = property on="Y steps/rev" class="DigNum (strict)"() -> ("Value"=w488:u32)  [unwired: 2 in, 2 out]
            n121 = To Double Precision Float(number=w488) -> (double precision float=w482:dbl)
            n122 = property on="Y Step SP" class="DigNum (strict)"() -> ("Maximum"=w493:dbl)  [unwired: 2 in, 2 out]
            n123 = property on="Y Step SP" class="DigNum (strict)"() -> ("Minimum"=w494:dbl)  [unwired: 2 in, 2 out]
            n124 = To Double Precision Float(number=w484) -> (double precision float=w483:dbl)
            n125 = To Double Precision Float(number=w486) -> (double precision float=w485:dbl)
            n126 = Subtract(x=w494, y=w483) -> (x-y=w495:dbl)
            n127 = Subtract(x=w493, y=w485) -> (x-y=w492:dbl)
            n128 = property on="Y Scan Length SP steps" class="DigNum (strict)"() -> ("Value"=w490:i32)  [unwired: 2 in, 2 out]
            n129 = property on="Y Scan Velocity SP steps/sec" class="DigNum (strict)"() -> ("Value"=w481:i32)  [unwired: 2 in, 2 out]
            n130 = To Double Precision Float(number=w490) -> (double precision float=w489:dbl)
            n131 = property on="Y Scan Length SP steps" class="DigNum (strict)"("Minimum"=w495) -> ()  [unwired: 2 in, 2 out]
            n132 = property on="Y Scan Length SP steps" class="DigNum (strict)"("Maximum"=w492) -> ()  [unwired: 2 in, 2 out]
            n133 = Divide(x=w489, y=w482) -> (x/y=w491:dbl)
            n134 = To Double Precision Float(number=w481) -> (double precision float=w480:dbl)
            n135 = property on="Y mm/rev" class="DigNum (strict)"() -> ("Value"=w487:dbl)  [unwired: 2 in, 2 out]
            n136 = Multiply(x=w491, y=w487) -> (x*y=w478:dbl)
            n137 = Divide(x=w480, y=w482) -> (x/y=w479:dbl)
            n138 = Multiply(x=w487, y=w479) -> (x*y=w477:dbl)
            n139 = property on="Y Scan length MV mm" class="DigNum (strict)"("Value"=w478) -> ()  [unwired: 2 in, 2 out]
            n140 = property on="Y Scan velocity MV mm/sec" class="DigNum (strict)"("Val(Sgnl)"=w477) -> ()  [unwired: 2 in, 2 out]
          }
        }
        n141 = flat-sequence {
          tunnel: [w237] -> w184
          tunnel: [w213] -> w183
          tunnel: [w226] -> w182
          tunnel: [w204] -> w181
          tunnel: w171 -> [w203]
          tunnel: w170 -> [w202]
          tunnel: w184 -> [w243]
          tunnel: [w243] -> w180
          tunnel: w183 -> [w242]
          tunnel: [w242] -> w179
          tunnel: w182 -> [w241]
          tunnel: [w241] -> w178
          tunnel: w181 -> [w238]
          tunnel: [w238] -> w177
          tunnel: w180 -> [w250]
          tunnel: [w251] -> w176
          tunnel: w179 -> [w253]
          tunnel: [w252] -> w175
          tunnel: w178 -> [w249]
          tunnel: [w248] -> w174
          tunnel: w177 -> [w248]
          tunnel: w176 -> [w263]
          tunnel: w175 -> [w264]
          tunnel: [w262] -> w173
          tunnel: w174 -> [w266]
          tunnel: [w261] -> w172
          tunnel: [w349] -> w168
          tunnel: w173 -> [w349]
          tunnel: w172 -> [w329]
          tunnel: [w329] -> w169
          frame #0 {
            w208 = 0.1 ("Delay Time (s)")
            n142 = property on="X Step SP" class="DigNum (strict)"() -> ("Maximum"=w228:dbl)  [unwired: 2 in, 2 out]
            n143 = property on="X Step SP" class="DigNum (strict)"() -> ("Minimum"=w230:dbl)  [unwired: 2 in, 2 out]
            n144 = property on="X steps/rev" class="DigNum (strict)"() -> ("Value"=w224:u32)  [unwired: 2 in, 2 out]
            n145 = property on="X offset mm" class="DigNum (strict)"() -> ("Value"=w220:dbl)  [unwired: 2 in, 2 out]
            n146 = call "mDrive Send Command.vi"("error in (no error)"=w202, "Extra"="P", "Command"=T2."Print Parameter", "VISA resource name"=w203) -> ("error out"=w232:errorcluster, "read buffer"=w236:string, "VISA resource name out"=w234:refnum<visa-resource-name>)  [unwired: 3 in]
            n147 = call "Time Delay12"("error in (no error)"=w232, "Delay Time (s)"=w208) -> ("error out"=w231:errorcluster)  [unwired: 9 in]
            n148 = Decimal String To Number(string=w236, offset=0) -> (number=w216:i32)  [unwired: 1 in, 1 out]
            n149 = To Long Integer(number=w216) -> (32bit integer=w218:i32)
            n150 = property on="X Step PV" class="DigNum (strict)"("Val(Sgnl)"=w218) -> ()  [unwired: 2 in, 2 out]
            n151 = To Long Integer(number=w228) -> (32bit integer=w227:i32)
            n152 = To Long Integer(number=w230) -> (32bit integer=w229:i32)
            n153 = call "mDrive Send Command.vi"("error in (no error)"=w231, "Extra"="MV", "Command"=T2."Print Parameter", "VISA resource name"=w234) -> ("error out"=w233:errorcluster, "read buffer"=w214:string, "VISA resource name out"=w237:refnum<visa-resource-name>)  [unwired: 3 in]
            n154 = call "Time Delay11"("error in (no error)"=w233, "Delay Time (s)"=w208) -> ("error out"=w213:errorcluster)  [unwired: 9 in]
            n155 = In Range and Coerce(upper limit=w227, x=w218, lower limit=w229) -> (In Range?=w226:bool)  [unwired: 1 out]
            n156 = To Double Precision Float(number=w218) -> (double precision float=w219:dbl)
            n157 = To Double Precision Float(number=w224) -> (double precision float=w225:dbl)
            n158 = Decimal String To Number(string=w214, offset=0 ("offset (0)")) -> (number=w207:i32)  [unwired: 1 in, 1 out]
            n159 = property on="X  in Range" class="Bool (strict)"("Val(Sgnl)"=w226) -> ()  [unwired: 2 in, 2 out]
            n160 = Divide(x=w219, y=w225) -> (x/y=w223:dbl)
            n161 = Number To Boolean Array(number=w207) -> (Boolean array=w206:bool[])
            n162 = property on="X mm/rev" class="DigNum (strict)"() -> ("Value"=w222:dbl)  [unwired: 2 in, 2 out]
            n163 = Index Array(array=w206, index=0) -> (element=w204:bool)
            n164 = property on="X  in Motion" class="Bool (strict)"("Val(Sgnl)"=w204) -> ()  [unwired: 2 in, 2 out]
            n165 = Multiply(x=w223, y=w222) -> (x*y=w221:dbl)
            n166 = Add(x=w221, y=w220) -> (x+y=w217:dbl)
            n167 = property on="X Position mm PV" class="DigNum (strict)"("Val(Sgnl)"=w217) -> ()  [unwired: 2 in, 2 out]
          }
          frame #1 {
            n168 = property on="X Scan" class="Bool (strict)"() -> ("Value"=w239:bool)  [unwired: 2 in, 2 out]
            n169 = Or(x=w238, y=w239) -> (x .or. y?=w240:bool)
            n170 = case shown="False" w240 {
              frame #0 {
                n171 = property on="X Go" class="Bool"("DisabledEnum"=T1."Enabled" ("Disabled")) -> ()  [unwired: 2 in, 2 out]
                n172 = property on="X Scan OK" class="Bool"("DisabledEnum"=T1."Enabled" ("Disabled")) -> ()  [unwired: 2 in, 2 out]
              }
              frame #1 {
                n173 = property on="X Go" class="Bool"("DisabledEnum"=T1."Disabled and Grayed Out" ("Disabled")) -> ()  [unwired: 2 in, 2 out]
                n174 = property on="X Scan set" class="Bool"("DisabledEnum"=T1."Disabled and Grayed Out" ("Disabled")) -> ()  [unwired: 2 in, 2 out]
              }
            }
          }
          frame #2 {
            n175 = case shown="False" w249 {
              tunnel: w250 -> [w256 w260]
              tunnel: [w257 w260] -> w251
              tunnel: [w258 w259] -> w252
              tunnel: w253 -> [w255 w259]
              frame #0 {
                n176 = call "mDrive Send Command.vi"("error in (no error)"=w255, "Command"=T2."Stop", "VISA resource name"=w256) -> ("error out"=w258:errorcluster, "VISA resource name out"=w257:refnum<visa-resource-name>)  [unwired: 4 in, 1 out]
              }
              frame #1 {
              }
            }
          }
          frame #3 {
            n177 = property on="X Backlash corr" class="Bool (strict)"() -> ("Value"=w267:bool)  [unwired: 2 in, 2 out]
            n178 = Implies(1:w266, 2:w267) -> (0:w265:bool)
            n179 = case shown="False" w265 {
              tunnel: w264 -> [w274 w327]
              tunnel: w263 -> [w273 w328]
              tunnel: [w272 w327] -> w262
              tunnel: [w271 w328] -> w261
              frame #0 {
                # "Backlash"
                n180 = flat-sequence {
                  tunnel: [w289] -> w286
                  tunnel: [w291] -> w285
                  tunnel: [w290] -> w284
                  tunnel: w274 -> [w288]
                  tunnel: w273 -> [w287]
                  tunnel: w286 -> [w299]
                  tunnel: [w299] -> w283
                  tunnel: w285 -> [w298]
                  tunnel: w284 -> [w297]
                  tunnel: [w296] -> w282
                  tunnel: [w295] -> w281
                  tunnel: [w294] -> w270
                  tunnel: w283 -> [w309]
                  tunnel: w282 -> [w308]
                  tunnel: w281 -> [w306]
                  tunnel: [w307] -> w280
                  tunnel: [w306] -> w279
                  tunnel: [w305] -> w276
                  tunnel: [w304] -> w275
                  tunnel: w270 -> [w304]
                  tunnel: w280 -> [w320]
                  tunnel: w279 -> [w313]
                  tunnel: [w320] -> w278
                  tunnel: [w319] -> w277
                  tunnel: w276 -> [w319]
                  tunnel: w275 -> [w315]
                  tunnel: [w314] -> w268
                  tunnel: w278 -> [w324]
                  tunnel: w277 -> [w323]
                  tunnel: [w322] -> w272
                  tunnel: [w321] -> w269
                  tunnel: w268 -> [w321]
                  tunnel: [w326] -> w271
                  tunnel: w269 -> [w326]
                  frame #0 {
                    n181 = property on="X Backlash steps/sec" class="DigNum (strict)"() -> ("Value"=w289:i32)  [unwired: 2 in, 2 out]
                    n182 = Number To Decimal String(number=w289) -> (decimal integer string=w292:string)  [unwired: 1 in]
                    n183 = call "mDrive Send Command.vi"("error in (no error)"=w288, "Extra"=w292, "Command"=T2."Max Velocity", "VISA resource name"=w287) -> ("error out"=w290:errorcluster, "VISA resource name out"=w291:refnum<visa-resource-name>)  [unwired: 3 in, 1 out]
                  }
                  frame #1 {
                    n184 = property on="X Backlash" class="DigNum (strict)"() -> ("Value"=w294:i32)  [unwired: 2 in, 2 out]
                    n185 = Number To Decimal String(number=w294) -> (decimal integer string=w300:string)  [unwired: 1 in]
                    n186 = call "mDrive Send Command.vi"("error in (no error)"=w297, "Extra"=w300, "Command"=T2."Move to Relative Position", "VISA resource name"=w298) -> ("error out"=w296:errorcluster, "VISA resource name out"=w295:refnum<visa-resource-name>)  [unwired: 3 in, 1 out]
                  }
                  frame #2 {
                    n187 = To Double Precision Float(number=w304) -> (double precision float=w302:dbl)
                    n188 = To Double Precision Float(number=w309) -> (double precision float=w311:dbl)
                    n189 = Absolute Value(x=w302) -> (abs(x)=w303:dbl)
                    n190 = Divide(x=w303, y=w311) -> (x/y=w312:dbl)
                    n191 = Add(x=w312, y=0.3) -> (x+y=w305:dbl)
                    n192 = call "Time Delay13"("error in (no error)"=w308, "Delay Time (s)"=w305) -> ("error out"=w307:errorcluster)  [unwired: 9 in]
                  }
                  frame #3 {
                    n193 = Negate(x=w315) -> (-x=w316:i32)
                    n194 = Number To Decimal String(number=w316) -> (decimal integer string=w317:string)  [unwired: 1 in]
                    n195 = call "mDrive Send Command.vi"("Extra"=w317, "Command"=T2."Move to Relative Position", "VISA resource name"=w313) -> ("VISA resource name out"=w314:refnum<visa-resource-name>)  [unwired: 4 in, 2 out]
                  }
                  frame #4 {
                    n196 = call "Time Delay14"("error in (no error)"=w324, "Delay Time (s)"=w323) -> ("error out"=w322:errorcluster)  [unwired: 9 in]
                  }
                  frame #5 {
                    n197 = property on="X Backlash corr" class="Bool (strict)"("Val(Sgnl)"=FALSE ("Value (Signaling)")) -> ()  [unwired: 2 in, 2 out]
                  }
                }
              }
              frame #1 {
              }
            }
          }
          frame #4 {
            n198 = property on="X Step PV" class="DigNum (strict)"() -> ("Value"=w337:i32)  [unwired: 2 in, 2 out]
            n199 = property on="X Step PV" class="DigNum (strict)"() -> ("Value"=w339:i32)  [unwired: 2 in, 2 out]
            n200 = property on="X steps/rev" class="DigNum (strict)"() -> ("Value"=w341:u32)  [unwired: 2 in, 2 out]
            n201 = To Double Precision Float(number=w341) -> (double precision float=w335:dbl)
            n202 = property on="X Step SP" class="DigNum (strict)"() -> ("Maximum"=w346:dbl)  [unwired: 2 in, 2 out]
            n203 = property on="X Step SP" class="DigNum (strict)"() -> ("Minimum"=w347:dbl)  [unwired: 2 in, 2 out]
            n204 = To Double Precision Float(number=w337) -> (double precision float=w336:dbl)
            n205 = To Double Precision Float(number=w339) -> (double precision float=w338:dbl)
            n206 = Subtract(x=w347, y=w336) -> (x-y=w348:dbl)
            n207 = Subtract(x=w346, y=w338) -> (x-y=w345:dbl)
            n208 = property on="X Scan Length SP steps" class="DigNum (strict)"() -> ("Value"=w334:i32)  [unwired: 2 in, 2 out]
            n209 = property on="X Scan Velocity SP steps/sec" class="DigNum (strict)"() -> ("Value"=w343:i32)  [unwired: 2 in, 2 out]
            n210 = To Double Precision Float(number=w334) -> (double precision float=w333:dbl)
            n211 = property on="X Scan Length SP steps" class="DigNum (strict)"("Minimum"=w348) -> ()  [unwired: 2 in, 2 out]
            n212 = property on="X Scan Length SP steps" class="DigNum (strict)"("Maximum"=w345) -> ()  [unwired: 2 in, 2 out]
            n213 = Divide(x=w333, y=w335) -> (x/y=w332:dbl)
            n214 = To Double Precision Float(number=w343) -> (double precision float=w342:dbl)
            n215 = property on="X mm/rev" class="DigNum (strict)"() -> ("Value"=w340:dbl)  [unwired: 2 in, 2 out]
            n216 = Divide(x=w342, y=w335) -> (x/y=w344:dbl)
            n217 = Multiply(x=w340, y=w332) -> (x*y=w330:dbl)
            n218 = Multiply(x=w344, y=w340) -> (x*y=w331:dbl)
            n219 = property on="X Scan length MV mm" class="DigNum (strict)"("Val(Sgnl)"=w330) -> ()  [unwired: 2 in, 2 out]
            n220 = property on="X Scan velocity MV mm/sec" class="DigNum (strict)"("Value"=w331) -> ()  [unwired: 2 in, 2 out]
          }
        }
      }
      event #1 {
        n221 = event-data() -> ()  [unwired: 1 in, 5 out]
        n222 = property on="X Step SP" class="DigNum (strict)"() -> ("Value"=w502:i32)  [unwired: 2 in, 2 out]
        n223 = property on="X steps/rev" class="DigNum (strict)"() -> ("Value"=w500:u32)  [unwired: 2 in, 2 out]
        n224 = property on="X offset mm" class="DigNum (strict)"() -> ("Value"=w498:dbl)  [unwired: 2 in, 2 out]
        n225 = To Double Precision Float(number=w502) -> (double precision float=w503:dbl)
        n226 = To Double Precision Float(number=w500) -> (double precision float=w506:dbl)
        n227 = Divide(x=w503, y=w506) -> (x/y=w505:dbl)
        n228 = property on="X mm/rev" class="DigNum (strict)"() -> ("Value"=w499:dbl)  [unwired: 2 in, 2 out]
        n229 = Multiply(x=w505, y=w499) -> (x*y=w504:dbl)
        n230 = Add(x=w504, y=w498) -> (x+y=w501:dbl)
        n231 = property on="X Position MV mm" class="DigNum (strict)"("Val(Sgnl)"=w501) -> ()  [unwired: 2 in, 2 out]
      }
      event #2 {
        n232 = event-data() -> ()  [unwired: 1 in, 5 out]
        n233 = property on="Y steps/rev" class="DigNum (strict)"() -> ("Value"=w509:u32)  [unwired: 2 in, 2 out]
        n234 = property on="Y offset mm" class="DigNum (strict)"() -> ("Value"=w507:dbl)  [unwired: 2 in, 2 out]
        n235 = property on="Reset Y Position mm" class="DigNum (strict)"() -> ("Value"=w515:dbl)  [unwired: 2 in, 2 out]
        n236 = Subtract(x=w515, y=w507) -> (x-y=w514:dbl)
        n237 = property on="Y mm/rev" class="DigNum (strict)"() -> ("Value"=w508:dbl)  [unwired: 2 in, 2 out]
        n238 = Divide(x=w514, y=w508) -> (x/y=w513:dbl)
        n239 = To Double Precision Float(number=w509) -> (double precision float=w512:dbl)
        n240 = Multiply(x=w513, y=w512) -> (x*y=w511:dbl)
        n241 = To Long Integer(number=w511) -> (32bit integer=w510:i32)
        n242 = property on="Reset Y Motor Steps" class="DigNum (strict)"("Val(Sgnl)"=w510) -> ()  [unwired: 2 in, 2 out]
      }
      event #3 {
        n243 = event-data() -> ()  [unwired: 1 in, 5 out]
        n244 = property on="Y Step SP" class="DigNum (strict)"() -> ("Value"=w520:i32)  [unwired: 2 in, 2 out]
        n245 = property on="Y steps/rev" class="DigNum (strict)"() -> ("Value"=w518:u32)  [unwired: 2 in, 2 out]
        n246 = property on="Y offset mm" class="DigNum (strict)"() -> ("Value"=w516:dbl)  [unwired: 2 in, 2 out]
        n247 = To Double Precision Float(number=w520) -> (double precision float=w521:dbl)
        n248 = To Double Precision Float(number=w518) -> (double precision float=w524:dbl)
        n249 = Divide(x=w521, y=w524) -> (x/y=w523:dbl)
        n250 = property on="Y mm/rev" class="DigNum (strict)"() -> ("Value"=w517:dbl)  [unwired: 2 in, 2 out]
        n251 = Multiply(x=w523, y=w517) -> (x*y=w522:dbl)
        n252 = Add(x=w522, y=w516) -> (x+y=w519:dbl)
        n253 = property on="Y Position MV mm" class="DigNum (strict)"("Val(Sgnl)"=w519) -> ()  [unwired: 2 in, 2 out]
      }
      event #4 {
        n254 = event-data() -> ()  [unwired: 1 in, 5 out]
        n255 = property on="X Step SP" class="DigNum (strict)"() -> ("Value"=w529:i32)  [unwired: 2 in, 2 out]
        n256 = property on="X steps/rev" class="DigNum (strict)"() -> ("Value"=w527:u32)  [unwired: 2 in, 2 out]
        n257 = property on="X offset mm" class="DigNum (strict)"() -> ("Value"=w525:dbl)  [unwired: 2 in, 2 out]
        n258 = To Double Precision Float(number=w529) -> (double precision float=w530:dbl)
        n259 = To Double Precision Float(number=w527) -> (double precision float=w533:dbl)
        n260 = Divide(x=w530, y=w533) -> (x/y=w532:dbl)
        n261 = property on="X mm/rev" class="DigNum (strict)"() -> ("Value"=w526:dbl)  [unwired: 2 in, 2 out]
        n262 = Multiply(x=w532, y=w526) -> (x*y=w531:dbl)
        n263 = Add(x=w531, y=w525) -> (x+y=w528:dbl)
        n264 = property on="X Position MV mm" class="DigNum (strict)"("Val(Sgnl)"=w528) -> ()  [unwired: 2 in, 2 out]
      }
      event #5 {
        n265 = event-data() -> ()  [unwired: 1 in, 5 out]
        n266 = property on="Y steps/rev" class="DigNum (strict)"() -> ("Value"=w535:u32)  [unwired: 2 in, 2 out]
        n267 = property on="Y Velocity SP step/sec" class="DigNum (strict)"() -> ("Value"=w537:i32)  [unwired: 2 in, 2 out]
        n268 = To Double Precision Float(number=w537) -> (double precision float=w538:dbl)
        n269 = To Double Precision Float(number=w535) -> (double precision float=w540:dbl)
        n270 = Divide(x=w538, y=w540) -> (x/y=w539:dbl)
        n271 = property on="Y mm/rev" class="DigNum (strict)"() -> ("Value"=w534:dbl)  [unwired: 2 in, 2 out]
        n272 = Multiply(x=w539, y=w534) -> (x*y=w536:dbl)
        n273 = property on="Y Velocity MV mm/sec" class="DigNum (strict)"("Val(Sgnl)"=w536) -> ()  [unwired: 2 in, 2 out]
      }
      event #6 {
        n274 = event-data() -> ()  [unwired: 1 in, 5 out]
        n275 = property on="X steps/rev" class="DigNum (strict)"() -> ("Value"=w542:u32)  [unwired: 2 in, 2 out]
        n276 = property on="X Velocity SP step/sec" class="DigNum (strict)"() -> ("Value"=w544:i32)  [unwired: 2 in, 2 out]
        n277 = To Double Precision Float(number=w544) -> (double precision float=w545:dbl)
        n278 = To Double Precision Float(number=w542) -> (double precision float=w547:dbl)
        n279 = Divide(x=w545, y=w547) -> (x/y=w546:dbl)
        n280 = property on="X mm/rev" class="DigNum (strict)"() -> ("Value"=w541:dbl)  [unwired: 2 in, 2 out]
        n281 = Multiply(x=w546, y=w541) -> (x*y=w543:dbl)
        n282 = property on="X Velocity MV mm/sec" class="DigNum (strict)"("Val(Sgnl)"=w543) -> ()  [unwired: 2 in, 2 out]
      }
      event #7 {
        n283 = event-data() -> ()  [unwired: 1 in, 7 out]
        n284 = flat-sequence {
          frame #0 {
            n285 = property on="Y steps/rev" class="DigNum (strict)"() -> ("Value"=w555:u32)  [unwired: 2 in, 2 out]
            n286 = property on="Y offset mm" class="DigNum (strict)"() -> ("Value"=w553:dbl)  [unwired: 2 in, 2 out]
            n287 = property on="Y Position SP mm" class="DigNum (strict)"() -> ("Value"=w552:dbl)  [unwired: 2 in, 2 out]
            n288 = Subtract(x=w552, y=w553) -> (x-y=w557:dbl)
            n289 = property on="Y mm/rev" class="DigNum (strict)"() -> ("Value"=w556:dbl)  [unwired: 2 in, 2 out]
            n290 = Divide(x=w557, y=w556) -> (x/y=w558:dbl)
            n291 = To Double Precision Float(number=w555) -> (double precision float=w559:dbl)
            n292 = Multiply(x=w558, y=w559) -> (x*y=w551:dbl)
            n293 = property on="Y Step SP" class="DigNum (strict)"() -> ("Maximum"=w549:dbl)  [unwired: 2 in, 2 out]
            n294 = property on="Y Step SP" class="DigNum (strict)"() -> ("Minimum"=w548:dbl)  [unwired: 2 in, 2 out]
            n295 = In Range and Coerce(upper limit=w549, x=w551, lower limit=w548) -> (coerced(x)=w550:dbl)  [unwired: 1 out]
            n296 = To Long Integer(number=w550) -> (32bit integer=w554:i32)
            n297 = property on="Y Step SP" class="DigNum (strict)"("Val(Sgnl)"=w554) -> ()  [unwired: 2 in, 2 out]
          }
          frame #1 {
            n298 = property on="Y steps/rev" class="DigNum (strict)"() -> ("Value"=w565:u32)  [unwired: 2 in, 2 out]
            n299 = To Double Precision Float(number=w565) -> (double precision float=w566:dbl)
            n300 = property on="Y Velocity SP step/sec" class="DigNum (strict)"() -> ("Minimum"=w560:dbl)  [unwired: 2 in, 2 out]
            n301 = property on="Y Velocity SP mm/sec" class="DigNum (strict)"() -> ("Value"=w567:dbl)  [unwired: 2 in, 2 out]
            n302 = property on="Y Velocity SP step/sec" class="DigNum (strict)"() -> ("Maximum"=w561:dbl)  [unwired: 2 in, 2 out]
            n303 = property on="Y mm/rev" class="DigNum (strict)"() -> ("Value"=w569:dbl)  [unwired: 2 in, 2 out]
            n304 = Divide(x=w567, y=w569) -> (x/y=w568:dbl)
            n305 = Multiply(x=w568, y=w566) -> (x*y=w563:dbl)
            n306 = In Range and Coerce(upper limit=w561, x=w563, lower limit=w560) -> (coerced(x)=w562:dbl)  [unwired: 1 out]
            n307 = To Long Integer(number=w562) -> (32bit integer=w564:i32)
            n308 = property on="Y Velocity SP step/sec" class="DigNum (strict)"("Val(Sgnl)"=w564) -> ()  [unwired: 2 in, 2 out]
          }
        }
      }
      event #8 {
        n309 = event-data() -> ()  [unwired: 1 in, 7 out]
        n310 = flat-sequence {
          frame #0 {
            n311 = property on="X steps/rev" class="DigNum (strict)"() -> ("Value"=w577:u32)  [unwired: 2 in, 2 out]
            n312 = property on="X offset mm" class="DigNum (strict)"() -> ("Value"=w575:dbl)  [unwired: 2 in, 2 out]
            n313 = property on="X Position SP mm" class="DigNum (strict)"() -> ("Value"=w574:dbl)  [unwired: 2 in, 2 out]
            n314 = Subtract(x=w574, y=w575) -> (x-y=w579:dbl)
            n315 = property on="X mm/rev" class="DigNum (strict)"() -> ("Value"=w578:dbl)  [unwired: 2 in, 2 out]
            n316 = Divide(x=w579, y=w578) -> (x/y=w580:dbl)
            n317 = To Double Precision Float(number=w577) -> (double precision float=w581:dbl)
            n318 = Multiply(x=w580, y=w581) -> (x*y=w573:dbl)
            n319 = property on="X Step SP" class="DigNum (strict)"() -> ("Maximum"=w571:dbl)  [unwired: 2 in, 2 out]
            n320 = property on="X Step SP" class="DigNum (strict)"() -> ("Minimum"=w570:dbl)  [unwired: 2 in, 2 out]
            n321 = In Range and Coerce(upper limit=w571, x=w573, lower limit=w570) -> (coerced(x)=w572:dbl)  [unwired: 1 out]
            n322 = To Long Integer(number=w572) -> (32bit integer=w576:i32)
            n323 = property on="X Step SP" class="DigNum (strict)"("Val(Sgnl)"=w576) -> ()  [unwired: 2 in, 2 out]
          }
          frame #1 {
            n324 = property on="X steps/rev" class="DigNum (strict)"() -> ("Value"=w587:u32)  [unwired: 2 in, 2 out]
            n325 = To Double Precision Float(number=w587) -> (double precision float=w588:dbl)
            n326 = property on="X Velocity SP step/sec" class="DigNum (strict)"() -> ("Minimum"=w582:dbl)  [unwired: 2 in, 2 out]
            n327 = property on="X Scan Velocity SP mm/sec" class="DigNum (strict)"() -> ("Value"=w589:dbl)  [unwired: 2 in, 2 out]
            n328 = property on="X Velocity SP step/sec" class="DigNum (strict)"() -> ("Maximum"=w583:dbl)  [unwired: 2 in, 2 out]
            n329 = property on="X mm/rev" class="DigNum (strict)"() -> ("Value"=w591:dbl)  [unwired: 2 in, 2 out]
            n330 = Divide(x=w589, y=w591) -> (x/y=w590:dbl)
            n331 = Multiply(x=w590, y=w588) -> (x*y=w585:dbl)
            n332 = In Range and Coerce(upper limit=w583, x=w585, lower limit=w582) -> (coerced(x)=w584:dbl)  [unwired: 1 out]
            n333 = To Long Integer(number=w584) -> (32bit integer=w586:i32)
            n334 = property on="X Velocity SP step/sec" class="DigNum (strict)"("Val(Sgnl)"=w586) -> ()  [unwired: 2 in, 2 out]
          }
        }
      }
      event #9 {
        n335 = event-data() -> ()  [unwired: 1 in, 7 out]
        n336 = flat-sequence {
          frame #0 {
            n337 = property on="Y steps/rev" class="DigNum (strict)"() -> ("Value"=w598:u32)  [unwired: 2 in, 2 out]
            n338 = property on="Y Scan Length SP mm" class="DigNum (strict)"() -> ("Value"=w596:dbl)  [unwired: 2 in, 2 out]
            n339 = property on="Y mm/rev" class="DigNum (strict)"() -> ("Value"=w599:dbl)  [unwired: 2 in, 2 out]
            n340 = Divide(x=w596, y=w599) -> (x/y=w600:dbl)
            n341 = To Double Precision Float(number=w598) -> (double precision float=w601:dbl)
            n342 = Multiply(x=w600, y=w601) -> (x*y=w595:dbl)
            n343 = property on="Y Step SP" class="DigNum (strict)"() -> ("Maximum"=w592:dbl)  [unwired: 2 in, 2 out]
            n344 = property on="Y Step SP" class="DigNum (strict)"() -> ("Minimum"=w593:dbl)  [unwired: 2 in, 2 out]
            n345 = In Range and Coerce(upper limit=w592, x=w595, lower limit=w593) -> (coerced(x)=w594:dbl)  [unwired: 1 out]
            n346 = To Long Integer(number=w594) -> (32bit integer=w597:i32)
            n347 = property on="Y Scan Length SP steps" class="DigNum (strict)"("Val(Sgnl)"=w597) -> ()  [unwired: 2 in, 2 out]
          }
          frame #1 {
            n348 = property on="Y steps/rev" class="DigNum (strict)"() -> ("Value"=w607:u32)  [unwired: 2 in, 2 out]
            n349 = To Double Precision Float(number=w607) -> (double precision float=w608:dbl)
            n350 = property on="Y Scan Velocity SP mm/sec" class="DigNum (strict)"() -> ("Value"=w609:dbl)  [unwired: 2 in, 2 out]
            n351 = property on="Y Scan Velocity SP steps/sec" class="DigNum (strict)"() -> ("Maximum"=w603:dbl)  [unwired: 2 in, 2 out]
            n352 = property on="Y Scan Velocity SP steps/sec" class="DigNum (strict)"() -> ("Minimum"=w602:dbl)  [unwired: 2 in, 2 out]
            n353 = property on="Y mm/rev" class="DigNum (strict)"() -> ("Value"=w611:dbl)  [unwired: 2 in, 2 out]
            n354 = Divide(x=w609, y=w611) -> (x/y=w610:dbl)
            n355 = Multiply(x=w610, y=w608) -> (x*y=w605:dbl)
            n356 = In Range and Coerce(upper limit=w603, x=w605, lower limit=w602) -> (coerced(x)=w604:dbl)  [unwired: 1 out]
            n357 = To Long Integer(number=w604) -> (32bit integer=w606:i32)
            n358 = property on="Y Scan Velocity SP steps/sec" class="DigNum (strict)"("Val(Sgnl)"=w606) -> ()  [unwired: 2 in, 2 out]
          }
        }
      }
      event #10 {
        n359 = event-data() -> ()  [unwired: 1 in, 7 out]
        n360 = flat-sequence {
          frame #0 {
            n361 = property on="X steps/rev" class="DigNum (strict)"() -> ("Value"=w618:u32)  [unwired: 2 in, 2 out]
            n362 = property on="X Scan Length SP mm" class="DigNum (strict)"() -> ("Value"=w616:dbl)  [unwired: 2 in, 2 out]
            n363 = property on="X mm/rev" class="DigNum (strict)"() -> ("Value"=w619:dbl)  [unwired: 2 in, 2 out]
            n364 = Divide(x=w616, y=w619) -> (x/y=w620:dbl)
            n365 = To Double Precision Float(number=w618) -> (double precision float=w621:dbl)
            n366 = Multiply(x=w620, y=w621) -> (x*y=w615:dbl)
            n367 = property on="X Step SP" class="DigNum (strict)"() -> ("Maximum"=w612:dbl)  [unwired: 2 in, 2 out]
            n368 = property on="X Step SP" class="DigNum (strict)"() -> ("Minimum"=w613:dbl)  [unwired: 2 in, 2 out]
            n369 = In Range and Coerce(upper limit=w612, x=w615, lower limit=w613) -> (coerced(x)=w614:dbl)  [unwired: 1 out]
            n370 = To Long Integer(number=w614) -> (32bit integer=w617:i32)
            n371 = property on="X Scan Length SP steps" class="DigNum (strict)"("Val(Sgnl)"=w617) -> ()  [unwired: 2 in, 2 out]
          }
          frame #1 {
            n372 = property on="X steps/rev" class="DigNum (strict)"() -> ("Value"=w627:u32)  [unwired: 2 in, 2 out]
            n373 = To Double Precision Float(number=w627) -> (double precision float=w628:dbl)
            n374 = property on="X Scan Velocity SP mm/sec" class="DigNum (strict)"() -> ("Value"=w629:dbl)  [unwired: 2 in, 2 out]
            n375 = property on="X Scan Velocity SP steps/sec" class="DigNum (strict)"() -> ("Maximum"=w623:dbl)  [unwired: 2 in, 2 out]
            n376 = property on="X Scan Velocity SP steps/sec" class="DigNum (strict)"() -> ("Minimum"=w622:dbl)  [unwired: 2 in, 2 out]
            n377 = property on="X mm/rev" class="DigNum (strict)"() -> ("Value"=w631:dbl)  [unwired: 2 in, 2 out]
            n378 = Divide(x=w629, y=w631) -> (x/y=w630:dbl)
            n379 = Multiply(x=w630, y=w628) -> (x*y=w625:dbl)
            n380 = In Range and Coerce(upper limit=w623, x=w625, lower limit=w622) -> (coerced(x)=w624:dbl)  [unwired: 1 out]
            n381 = To Long Integer(number=w624) -> (32bit integer=w626:i32)
            n382 = property on="X Scan Velocity SP steps/sec" class="DigNum (strict)"("Val(Sgnl)"=w626) -> ()  [unwired: 2 in, 2 out]
          }
        }
      }
      event #11 {
        n383 = event-data() -> ()  [unwired: 1 in, 7 out]
        n384 = flat-sequence {
          tunnel: w636 -> [w646]
          tunnel: w637 -> [w647]
          tunnel: [w647] -> w633
          tunnel: [w646] -> w632
          tunnel: [w650] -> w635
          tunnel: [w649] -> w634
          tunnel: w633 -> [w652]
          tunnel: w632 -> [w651]
          tunnel: [w670] -> w639
          tunnel: [w669] -> w638
          tunnel: w635 -> [w668]
          tunnel: w634 -> [w667]
          tunnel: [w677] -> w641
          tunnel: [w676] -> w640
          tunnel: w639 -> [w675]
          tunnel: w638 -> [w674]
          tunnel: [w683] -> w642
          tunnel: [w684] -> w643
          tunnel: w641 -> [w684]
          tunnel: w640 -> [w682]
          frame #0 {
            n385 = property on="Scan Go" class="Bool"("DisabledEnum"=T1."Disabled and Grayed Out" ("Disabled")) -> ()  [unwired: 2 in, 2 out]
            n386 = property on="Y Go" class="Bool"("DisabledEnum"=T1."Disabled and Grayed Out" ("Disabled")) -> ()  [unwired: 2 in, 2 out]
          }
          frame #1 {
            n387 = property on="Y Step SP" class="DigNum (strict)"() -> ("Value"=w660:i32)  [unwired: 2 in, 2 out]
            n388 = property on="Y Step PV" class="DigNum (strict)"() -> ("Value"=w659:i32)  [unwired: 2 in, 2 out]
            n389 = property on="Y Backlash" class="DigNum (strict)"() -> ("Value"=w648:i32)  [unwired: 2 in, 2 out]
            n390 = Subtract(x=w660, y=w659) -> (x-y=w658:i32)
            n391 = Sign(1:w658) -> (0:w657:i32)
            n392 = Sign(1:w648) -> (0:w656:i32)
            n393 = Multiply(x=w657, y=w656) -> (x*y=w655:i32)
            n394 = Equal?(x=w655, y=1) -> (x = y?=w653:bool)
            n395 = case shown="False" w653 {
              tunnel: w652 -> [w663 w665]
              tunnel: w651 -> [w662 w664]
              tunnel: [w662 w664] -> w650
              tunnel: [w663 w665] -> w649
              frame #0 {
                n396 = property on="Y Backlash corr" class="Bool (strict)"("Val(Sgnl)"=FALSE ("Value (Signaling)")) -> ()  [unwired: 2 in, 2 out]
              }
              frame #1 {
                n397 = property on="Y Backlash corr" class="Bool (strict)"("Val(Sgnl)"=TRUE ("Value (Signaling)")) -> ()  [unwired: 2 in, 2 out]
              }
            }
          }
          frame #2 {
            # "Velocity Setting"
            n398 = property on="Y Velocity SP step/sec" class="DigNum (strict)"() -> ("Value"=w671:i32)  [unwired: 2 in, 2 out]
            n399 = Number To Decimal String(number=w671) -> (decimal integer string=w672:string)  [unwired: 1 in]
            n400 = call "mDrive Send Command.vi"("error in (no error)"=w668, "Extra"=w672, "Command"=T2."Max Velocity", "VISA resource name"=w667) -> ("error out"=w669:errorcluster, "VISA resource name out"=w670:refnum<visa-resource-name>)  [unwired: 3 in, 1 out]
          }
          frame #3 {
            # "Move to Abs Position"
            n401 = property on="Y Step SP" class="DigNum (strict)"() -> ("Value"=w680:i32)  [unwired: 2 in, 2 out]
            n402 = Number To Decimal String(number=w680) -> (decimal integer string=w679:string)  [unwired: 1 in]
            n403 = call "mDrive Send Command.vi"("error in (no error)"=w674, "Extra"=w679, "Command"=T2."Move to Absolute Position", "VISA resource name"=w675) -> ("error out"=w676:errorcluster, "VISA resource name out"=w677:refnum<visa-resource-name>)  [unwired: 3 in, 1 out]
          }
          frame #4 {
            n404 = call "Time Delay"("error in (no error)"=w682, "Delay Time (s)"=0.1) -> ("error out"=w683:errorcluster)  [unwired: 9 in]
          }
        }
      }
      event #12 {
        n405 = event-data() -> ()  [unwired: 1 in, 7 out]
        n406 = flat-sequence {
          tunnel: [w698] -> w690
          tunnel: [w697] -> w689
          tunnel: w688 -> [w698]
          tunnel: w687 -> [w697]
          tunnel: [w703] -> w692
          tunnel: [w702] -> w691
          tunnel: w690 -> [w705]
          tunnel: w689 -> [w704]
          tunnel: [w723] -> w694
          tunnel: [w722] -> w693
          tunnel: w692 -> [w721]
          tunnel: w691 -> [w720]
          tunnel: [w730] -> w696
          tunnel: [w729] -> w695
          tunnel: w694 -> [w728]
          tunnel: w693 -> [w727]
          tunnel: [w736] -> w685
          tunnel: [w737] -> w686
          tunnel: w696 -> [w737]
          tunnel: w695 -> [w735]
          frame #0 {
            n407 = property on="Scan Go" class="Bool"("DisabledEnum"=T1."Disabled and Grayed Out" ("Disabled")) -> ()  [unwired: 2 in, 2 out]
            n408 = property on="X Go" class="Bool"("DisabledEnum"=T1."Disabled and Grayed Out" ("Disabled")) -> ()  [unwired: 2 in, 2 out]
          }
          frame #1 {
            n409 = property on="X Step SP" class="DigNum (strict)"() -> ("Value"=w713:i32)  [unwired: 2 in, 2 out]
            n410 = property on="X Step PV" class="DigNum (strict)"() -> ("Value"=w712:i32)  [unwired: 2 in, 2 out]
            n411 = property on="X Backlash" class="DigNum (strict)"() -> ("Value"=w701:i32)  [unwired: 2 in, 2 out]
            n412 = Subtract(x=w713, y=w712) -> (x-y=w711:i32)
            n413 = Sign(1:w711) -> (0:w710:i32)
            n414 = Sign(1:w701) -> (0:w709:i32)
            n415 = Multiply(x=w710, y=w709) -> (x*y=w708:i32)
            n416 = Equal?(x=w708, y=1) -> (x = y?=w706:bool)
            n417 = case shown="False" w706 {
              tunnel: w705 -> [w716 w718]
              tunnel: w704 -> [w715 w717]
              tunnel: [w715 w717] -> w703
              tunnel: [w716 w718] -> w702
              frame #0 {
                n418 = property on="X Backlash corr" class="Bool (strict)"("Val(Sgnl)"=FALSE ("Value (Signaling)")) -> ()  [unwired: 2 in, 2 out]
              }
              frame #1 {
                n419 = property on="Y Backlash corr" class="Bool (strict)"("Val(Sgnl)"=TRUE ("Value (Signaling)")) -> ()  [unwired: 2 in, 2 out]
              }
            }
          }
          frame #2 {
            # "Velocity Setting"
            n420 = property on="X Scan Velocity SP steps/sec" class="DigNum (strict)"() -> ("Value"=w724:i32)  [unwired: 2 in, 2 out]
            n421 = Number To Decimal String(number=w724) -> (decimal integer string=w725:string)  [unwired: 1 in]
            n422 = call "mDrive Send Command.vi"("error in (no error)"=w721, "Extra"=w725, "Command"=T2."Max Velocity", "VISA resource name"=w720) -> ("error out"=w722:errorcluster, "VISA resource name out"=w723:refnum<visa-resource-name>)  [unwired: 3 in, 1 out]
          }
          frame #3 {
            # "Move to Abs Position"
            n423 = property on="X Step SP" class="DigNum (strict)"() -> ("Value"=w733:i32)  [unwired: 2 in, 2 out]
            n424 = Number To Decimal String(number=w733) -> (decimal integer string=w732:string)  [unwired: 1 in]
            n425 = call "mDrive Send Command.vi"("error in (no error)"=w727, "Extra"=w732, "Command"=T2."Move to Absolute Position", "VISA resource name"=w728) -> ("error out"=w729:errorcluster, "VISA resource name out"=w730:refnum<visa-resource-name>)  [unwired: 3 in, 1 out]
          }
          frame #4 {
            n426 = call "Time Delay15"("error in (no error)"=w735, "Delay Time (s)"=0.1) -> ("error out"=w736:errorcluster)  [unwired: 9 in]
          }
        }
      }
      event #13 {
        n427 = event-data() -> ()  [unwired: 1 in, 7 out]
        n428 = flat-sequence {
          tunnel: [w753] -> w745
          tunnel: [w751] -> w744
          tunnel: w743 -> [w747]
          tunnel: w742 -> [w746]
          tunnel: w745 -> [w768]
          tunnel: w744 -> [w767]
          tunnel: [w768] -> w739
          tunnel: [w767] -> w738
          tunnel: [w771] -> w740
          tunnel: [w772] -> w741
          tunnel: w739 -> [w772]
          tunnel: w738 -> [w771]
          frame #0 {
            # "VELOCITY"
            n429 = property on="X Scan Velocity SP steps/sec" class="DigNum (strict)"() -> ("Value"=w754:i32)  [unwired: 2 in, 2 out]
            n430 = Number To Decimal String(number=w754) -> (decimal integer string=w755:string)  [unwired: 1 in]
            n431 = call "mDrive Send Command.vi"("error in (no error)"=w746, "Extra"=w755, "Command"=T2."Max Velocity", "VISA resource name"=w747) -> ("error out"=w756:errorcluster, "VISA resource name out"=w761:refnum<visa-resource-name>)  [unwired: 3 in, 1 out]
            n432 = call "Time Delay9"("error in (no error)"=w756) -> ("error out"=w759:errorcluster)  [unwired: 10 in]
            n433 = call "mDrive Send Command.vi"("error in (no error)"=w759, "Extra"="VM", "Command"=T2."Print Parameter", "VISA resource name"=w761) -> ("error out"=w752:errorcluster, "read buffer"=w757:string, "VISA resource name out"=w753:refnum<visa-resource-name>)  [unwired: 3 in]
            n434 = call "Time Delay10"("error in (no error)"=w752) -> ("error out"=w751:errorcluster)  [unwired: 10 in]
            n435 = Decimal String To Number(string=w757, offset=0) -> (number=w760:i32)  [unwired: 1 in, 1 out]
            n436 = property on="X scan steps/sec MV step/sec" class="DigNum (strict)"("Val(Sgnl)"=w760) -> ()  [unwired: 2 in, 2 out]
          }
          frame #1 {
            n437 = property on="X Scan" class="Bool (strict)"("Val(Sgnl)"=TRUE ("Slew Ready 2")) -> ()  [unwired: 2 in, 2 out]
            n438 = property on="Scan Go" class="Bool"("DisabledEnum"=T1."Enabled" ("Disabled")) -> ()  [unwired: 2 in, 2 out]
            n439 = property on="Scan Cancel" class="Bool"("DisabledEnum"=T1."Enabled" ("Disabled")) -> ()  [unwired: 2 in, 2 out]
            n440 = property on="X Scan Velocity SP steps/sec" class="DigNum (strict)"("DisabledEnum"=T1."Disabled and Grayed Out" ("Disabled")) -> ()  [unwired: 2 in, 2 out]
            n441 = property on="X Scan Length SP steps" class="DigNum (strict)"("DisabledEnum"=T1."Disabled and Grayed Out" ("Disabled")) -> ()  [unwired: 2 in, 2 out]
          }
          frame #2 {
            n442 = property on="X Go" class="Bool"("DisabledEnum"=T1."Disabled and Grayed Out" ("Disabled")) -> ()  [unwired: 2 in, 2 out]
            n443 = property on="Y Go" class="Bool"("DisabledEnum"=T1."Disabled and Grayed Out" ("Disabled")) -> ()  [unwired: 2 in, 2 out]
          }
        }
      }
      event #14 {
        n444 = event-data() -> ()  [unwired: 1 in, 7 out]
        n445 = flat-sequence {
          tunnel: w780 -> [w790]
          tunnel: w779 -> [w789]
          tunnel: [w786] -> w777
          tunnel: [w784] -> w776
          tunnel: w777 -> [w803]
          tunnel: w776 -> [w802]
          tunnel: [w803] -> w774
          tunnel: [w802] -> w773
          tunnel: [w806] -> w778
          tunnel: [w807] -> w775
          tunnel: w774 -> [w807]
          tunnel: w773 -> [w806]
          frame #0 {
            # "VELOCITY"
            n446 = property on="Y Scan Velocity SP steps/sec" class="DigNum (strict)"() -> ("Value"=w787:i32)  [unwired: 2 in, 2 out]
            n447 = Number To Decimal String(number=w787) -> (decimal integer string=w788:string)  [unwired: 1 in]
            n448 = call "mDrive Send Command.vi"("error in (no error)"=w790, "Extra"=w788, "Command"=T2."Max Velocity", "VISA resource name"=w789) -> ("error out"=w791:errorcluster, "VISA resource name out"=w796:refnum<visa-resource-name>)  [unwired: 3 in, 1 out]
            n449 = call "Time Delay5"("error in (no error)"=w791) -> ("error out"=w794:errorcluster)  [unwired: 10 in]
            n450 = call "mDrive Send Command.vi"("error in (no error)"=w794, "Extra"="VM", "Command"=T2."Print Parameter", "VISA resource name"=w796) -> ("error out"=w785:errorcluster, "read buffer"=w792:string, "VISA resource name out"=w786:refnum<visa-resource-name>)  [unwired: 3 in]
            n451 = call "Time Delay6"("error in (no error)"=w785) -> ("error out"=w784:errorcluster)  [unwired: 10 in]
            n452 = Decimal String To Number(string=w792, offset=0) -> (number=w795:i32)  [unwired: 1 in, 1 out]
            n453 = property on="Y scan steps/sec MV step/sec" class="DigNum (strict)"("Val(Sgnl)"=w795) -> ()  [unwired: 2 in, 2 out]
          }
          frame #1 {
            n454 = property on="Y Scan" class="Bool (strict)"("Val(Sgnl)"=TRUE ("Slew Ready 2")) -> ()  [unwired: 2 in, 2 out]
            n455 = property on="Scan Go" class="Bool"("DisabledEnum"=T1."Enabled" ("Disabled")) -> ()  [unwired: 2 in, 2 out]
            n456 = property on="Scan Cancel" class="Bool"("DisabledEnum"=T1."Enabled" ("Disabled")) -> ()  [unwired: 2 in, 2 out]
            n457 = property on="Y Scan Velocity SP steps/sec" class="DigNum (strict)"("DisabledEnum"=T1."Disabled and Grayed Out" ("Disabled")) -> ()  [unwired: 2 in, 2 out]
            n458 = property on="Y Scan Length SP steps" class="DigNum (strict)"("DisabledEnum"=T1."Disabled and Grayed Out" ("Disabled")) -> ()  [unwired: 2 in, 2 out]
          }
          frame #2 {
            n459 = property on="Y Go" class="Bool"("DisabledEnum"=T1."Disabled and Grayed Out" ("Disabled")) -> ()  [unwired: 2 in, 2 out]
            n460 = property on="X Go" class="Bool"("DisabledEnum"=T1."Disabled and Grayed Out" ("Disabled")) -> ()  [unwired: 2 in, 2 out]
          }
        }
      }
      event #15 {
        n461 = event-data() -> ()  [unwired: 1 in, 4 out]
        n462 = event-data() -> ()  [unwired: 3 in, 1 out]
      }
      event #16 {
        n463 = event-data() -> ()  [unwired: 1 in, 7 out]
        n464 = call "mDrive Send Command.vi"("error in (no error)"=w819, "Command"=T2."Stop", "VISA resource name"=w820) -> ("error out"=w817:errorcluster, "VISA resource name out"=w818:refnum<visa-resource-name>)  [unwired: 4 in, 1 out]
        n465 = call "mDrive Send Command.vi"("error in (no error)"=w811, "Command"=T2."Stop", "VISA resource name"=w812) -> ("error out"=w813:errorcluster, "VISA resource name out"=w814:refnum<visa-resource-name>)  [unwired: 4 in, 1 out]
      }
      event #17 {
        n466 = event-data() -> ()  [unwired: 1 in, 7 out]
        n467 = flat-sequence {
          tunnel: w832 -> [w850]
          tunnel: w831 -> [w849]
          tunnel: [w852] -> w828
          tunnel: [w851] -> w827
          tunnel: [w859] -> w833
          tunnel: [w860] -> w834
          tunnel: w828 -> [w860]
          tunnel: w827 -> [w859]
          frame #0 {
            n468 = call "mDrive Send Command.vi"("error in (no error)"=w849, "Command"=T2."Stop", "VISA resource name"=w850) -> ("error out"=w851:errorcluster, "VISA resource name out"=w852:refnum<visa-resource-name>)  [unwired: 4 in, 1 out]
          }
          frame #1 {
            n469 = property on="Y Scan" class="Bool (strict)"("Value"=FALSE ("Slew Ready")) -> ()  [unwired: 2 in, 2 out]
            n470 = property on="Y Scan OK" class="Bool"("DisabledEnum"=T1."Enabled" ("Disabled")) -> ()  [unwired: 2 in, 2 out]
            n471 = property on="Y Scan Length SP steps" class="DigNum (strict)"("DisabledEnum"=T1."Enabled" ("Disabled")) -> ()  [unwired: 2 in, 2 out]
            n472 = property on="Y Scan OK" class="Bool"("DisabledEnum"=T1."Enabled" ("Disabled")) -> ()  [unwired: 2 in, 2 out]
            n473 = property on="Y Scan Velocity SP steps/sec" class="DigNum (strict)"("DisabledEnum"=T1."Enabled" ("Disabled")) -> ()  [unwired: 2 in, 2 out]
            n474 = property on="Y Go" class="Bool"("DisabledEnum"=T1."Enabled" ("Disabled")) -> ()  [unwired: 2 in, 2 out]
          }
        }
        n475 = flat-sequence {
          tunnel: w824 -> [w837]
          tunnel: w823 -> [w836]
          tunnel: [w839] -> w826
          tunnel: [w838] -> w825
          tunnel: [w846] -> w821
          tunnel: [w847] -> w822
          tunnel: w826 -> [w847]
          tunnel: w825 -> [w846]
          frame #0 {
            n476 = call "mDrive Send Command.vi"("error in (no error)"=w836, "Command"=T2."Stop", "VISA resource name"=w837) -> ("error out"=w838:errorcluster, "VISA resource name out"=w839:refnum<visa-resource-name>)  [unwired: 4 in, 1 out]
          }
          frame #1 {
            n477 = property on="X Scan" class="Bool (strict)"("Value"=FALSE ("Slew Ready")) -> ()  [unwired: 2 in, 2 out]
            n478 = property on="X Scan set" class="Bool"("DisabledEnum"=T1."Enabled" ("Disabled")) -> ()  [unwired: 2 in, 2 out]
            n479 = property on="X Scan Velocity SP steps/sec" class="DigNum (strict)"("DisabledEnum"=T1."Enabled" ("Disabled")) -> ()  [unwired: 2 in, 2 out]
            n480 = property on="X Scan Length SP steps" class="DigNum (strict)"("DisabledEnum"=T1."Enabled" ("Disabled")) -> ()  [unwired: 2 in, 2 out]
            n481 = property on="X Go" class="Bool"("DisabledEnum"=T1."Enabled" ("Disabled")) -> ()  [unwired: 2 in, 2 out]
            n482 = property on="X Scan OK" class="Bool"("DisabledEnum"=T1."Enabled" ("Disabled")) -> ()  [unwired: 2 in, 2 out]
          }
        }
        n483 = property on="Scan Go" class="Bool"("DisabledEnum"=T1."Disabled and Grayed Out" ("Disabled")) -> ()  [unwired: 2 in, 2 out]
        n484 = property on="Scan Cancel" class="Bool"("DisabledEnum"=T1."Disabled and Grayed Out" ("Disabled")) -> ()  [unwired: 2 in, 2 out]
      }
      event #18 {
        n485 = event-data() -> ()  [unwired: 1 in, 7 out]
        n486 = property on="Y Scan" class="Bool (strict)"() -> ("Value"=w864:bool)  [unwired: 2 in, 2 out]
        n487 = flat-sequence {
          tunnel: w877 -> [w880]
          tunnel: w876 -> [w881]
          tunnel: [w881] -> w873
          tunnel: [w880] -> w872
          tunnel: [w879] -> w871
          tunnel: w864 -> [w878]
          tunnel: [w878] -> w863
          tunnel: w873 -> [w892]
          tunnel: [w894] -> w868
          tunnel: w872 -> [w891]
          tunnel: [w893] -> w866
          tunnel: w871 -> [w890]
          tunnel: w863 -> [w889]
          tunnel: [w889] -> w861
          tunnel: w868 -> [w905]
          tunnel: [w905] -> w867
          tunnel: w866 -> [w904]
          tunnel: [w904] -> w865
          tunnel: [w902] -> w862
          tunnel: w861 -> [w902]
          tunnel: w867 -> [w910]
          tunnel: [w908] -> w870
          tunnel: w865 -> [w909]
          tunnel: [w907] -> w869
          tunnel: w862 -> [w906]
          tunnel: w870 -> [w926]
          tunnel: w869 -> [w925]
          tunnel: [w926] -> w875
          tunnel: [w925] -> w874
          frame #0 {
            n488 = case shown="True" w878 {
              tunnel: ["" w883] -> w879
              frame #0 {
              }
              frame #1 {
                n489 = property on="Y Scan Length SP steps" class="DigNum (strict)"() -> ("Value"=w888:i32)  [unwired: 2 in, 2 out]
                n490 = Number To Decimal String(number=w888) -> (decimal integer string=w885:string)  [unwired: 1 in]
                n491 = call <vilib>:"Space Constant.vi"() -> ("String"=w886:string)
                n492 = Concatenate Strings("MR", w886, w885, "\r") -> (w883:string)
              }
            }
          }
          frame #1 {
            n493 = case shown="True" w889 {
              tunnel: [w896 w901] -> w894
              tunnel: [w895 w900] -> w893
              tunnel: w892 -> [w896 w899]
              tunnel: w891 -> [w895 w898]
              tunnel: w890 -> [_ w897]
              frame #0 {
              }
              frame #1 {
                n494 = VISA Write(VISA resource name=w899, write buffer=w897, error in (no error)=w898) -> (VISA resource name out=w901:refnum<visa-resource-name>, error out=w900:errorcluster)  [unwired: 1 out]
              }
            }
          }
          frame #2 {
            n495 = call "Time Delay7"("Delay Time (s)"=0.1) -> ()  [unwired: 10 in, 1 out]
          }
          frame #3 {
            n496 = case shown="True" w906 {
              tunnel: w910 -> [w912 w916]
              tunnel: w909 -> [w911 w915]
              tunnel: [w912 w914] -> w908
              tunnel: [w911 w913] -> w907
              frame #0 {
              }
              frame #1 {
                n497 = property class="Instr"(reference=w916, error in=w915) -> (reference out=w918:refnum<visa-resource-name>, error out=w917:errorcluster, "Serial Settings:Number of Bytes at Serial Port"=w919:u32)
                n498 = VISA Read(VISA resource name=w918, byte count=w919, error in (no error)=w917) -> (VISA resource name out=w914:refnum<visa-resource-name>, error out=w913:errorcluster)  [unwired: 2 out]
              }
            }
          }
          frame #4 {
            n499 = property on="Y Scan" class="Bool (strict)"("Val(Sgnl)"=FALSE ("Slew Ready 2")) -> ()  [unwired: 2 in, 2 out]
            n500 = property on="Slew Velocity" class="DigNum (strict)"("DisabledEnum"=T1."Enabled" ("Disabled")) -> ()  [unwired: 2 in, 2 out]
            n501 = property on="Y Scan Length SP steps" class="DigNum (strict)"("DisabledEnum"=T1."Enabled" ("Disabled")) -> ()  [unwired: 2 in, 2 out]
            n502 = property on="Scan Go" class="Bool"("DisabledEnum"=T1."Disabled and Grayed Out" ("Disabled")) -> ()  [unwired: 2 in, 2 out]
            n503 = property on="Scan Cancel" class="Bool"("DisabledEnum"=T1."Disabled and Grayed Out" ("Disabled")) -> ()  [unwired: 2 in, 2 out]
          }
        }
      }
      event #19 {
        n504 = event-data() -> ()  [unwired: 1 in, 7 out]
        n505 = flat-sequence {
          tunnel: w934 -> [w945]
          tunnel: w933 -> [w944]
          tunnel: [w943] -> w932
          tunnel: [w942] -> w931
          frame #0 {
            n506 = property on="Reset Y Motor Steps" class="DigNum (strict)"() -> ("Value"=w946:i32)  [unwired: 2 in, 2 out]
            n507 = Number To Decimal String(number=w946) -> (decimal integer string=w947:string)  [unwired: 1 in]
            n508 = call "mDrive Send Command.vi"("error in (no error)"=w944, "Extra"=w947, "Command"=T2."Set Current Position", "VISA resource name"=w945) -> ("error out"=w942:errorcluster, "VISA resource name out"=w943:refnum<visa-resource-name>)  [unwired: 3 in, 1 out]
          }
        }
        n509 = flat-sequence {
          tunnel: [w935] -> w928
          tunnel: w929 -> [w938]
          tunnel: [w937] -> _
          tunnel: [w936] -> w927
          tunnel: w930 -> [w935]
          frame #0 {
            n510 = property on="Reset X Motor Steps" class="DigNum (strict)"() -> ("Value"=w939:i32)  [unwired: 2 in, 2 out]
            n511 = Number To Decimal String(number=w939) -> (decimal integer string=w940:string)  [unwired: 1 in]
            n512 = call "mDrive Send Command.vi"("error in (no error)"=w938, "Extra"=w940, "Command"=T2."Set Current Position", "VISA resource name"=w935) -> ("error out"=w936:errorcluster, "VISA resource name out"=w937:refnum<visa-resource-name>)  [unwired: 3 in, 1 out]
          }
        }
      }
    }
  }
  n513 = To Long Integer(number=w67) -> (32bit integer=w73:i32)
  n514 = To Long Integer(number=w23) -> (32bit integer=w27:i32)
  n515 = property on="Y Step SP" class="DigNum (strict)"("Maximum"=w68) -> ()  [unwired: 2 in, 2 out]
  n516 = property on="Y Step SP" class="DigNum (strict)"("Val(Sgnl)"=w73) -> ()  [unwired: 2 in, 2 out]
  n517 = property on="Y Step SP" class="DigNum (strict)"("Minimum"=w69) -> ()  [unwired: 2 in, 2 out]
  n518 = property on="X Step SP" class="DigNum (strict)"("Maximum"=w24) -> ()  [unwired: 2 in, 2 out]
  n519 = property on="X Step SP" class="DigNum (strict)"("Val(Sgnl)"=w27) -> ()  [unwired: 2 in, 2 out]
  n520 = property on="X Step SP" class="DigNum (strict)"("Minimum"=w25) -> ()  [unwired: 2 in, 2 out]
  n521 = In Range and Coerce(upper limit=w68, x=w73, lower limit=w69) -> (In Range?=w70:bool)  [unwired: 1 out]
  n522 = In Range and Coerce(upper limit=w24, x=w27, lower limit=w25) -> (In Range?=w26:bool)  [unwired: 1 out]
  n523 = property on="Y in Range" class="Bool (strict)"("Val(Sgnl)"=w70) -> ()  [unwired: 2 in, 2 out]
  n524 = property on="X  in Range" class="Bool (strict)"("Val(Sgnl)"=w26) -> ()  [unwired: 2 in, 2 out]
  n525 = flat-sequence {
    tunnel: w72 -> [w953]
    tunnel: w71 -> [w950]
    frame #0 {
      n526 = call "mDrive Send Command.vi"("error in (no error)"=w950, "Command"=T2."Stop", "VISA resource name"=w953) -> ("error out"=w951:errorcluster, "VISA resource name out"=w952:refnum<visa-resource-name>)  [unwired: 4 in, 1 out]
      n527 = VISA Close(VISA resource name=w952, error in (no error)=w951) -> ()  [unwired: 1 out]
    }
  }
  n528 = flat-sequence {
    tunnel: w2 -> [w958]
    tunnel: w1 -> [w955]
    frame #0 {
      n529 = call "mDrive Send Command.vi"("error in (no error)"=w955, "Command"=T2."Stop", "VISA resource name"=w958) -> ("error out"=w956:errorcluster, "VISA resource name out"=w957:refnum<visa-resource-name>)  [unwired: 4 in, 1 out]
      n530 = VISA Close(VISA resource name=w957, error in (no error)=w956) -> ()  [unwired: 1 out]
    }
  }
  "Y COM PORT" <- w76
  "Y MINPOS" <- w69
  "Y MAXPOS" <- w68
  "Y steps/rev" <- w46
  "Y mm/rev" <- w49
  "Y offset mm" <- 0.0 ("offset")
  "Y Run Current %" <- 60 ("Run Current %")
  "Y Holding Current %" <- 25 ("Holding Current %")
  "Y Backlash" <- -5120 ("Backlash2")
  "Y Backlash steps/sec" <- 25600 ("Value (Signaling)")
  "X COM PORT" <- w28
  "X MINPOS" <- w25
  "X MAXPOS" <- w24
  "X steps/rev" <- w10
  "X mm/rev" <- w13
  "X offset mm" <- 0.0 ("offset")
  "X Run Current %" <- 60 ("Run Current %")
  "X Holding Current %" <- 25 ("Holding Current %")
  "X Backlash" <- -5120 ("Backlash2")
  "X Backlash steps/sec" <- 25600 ("Value (Signaling)")
